vi "数字量输出配置.vi"() -> ()   [LabVIEW 2010]
panel:
  in  "保持输出":bool
  in  "同步_A2":i32
  in  "同步_A1":i32
  in  "数组_输入值":enum16{"0", "1"}[][](array[ring])
  in  "数组_选择?":bool[][](array[boolean])
  in  "btn_置1_5":bool
  in  "btn_置1_4":bool
  in  "btn_置1_3":bool
  in  "btn_置1_2":bool
  in  "btn_全选_5":bool
  in  "btn_全选_4":bool
  in  "btn_全选_3":bool
  in  "btn_全选_2":bool
  in  "btn_置1_1":bool
  in  "btn_全选_1":bool
  in  "CAN端口":u16
  out "light_80":bool
  out "light_79":bool
  out "light_78":bool
  out "light_77":bool
  out "light_76":bool
  out "light_75":bool
  out "light_74":bool
  out "light_73":bool
  out "light_72":bool
  out "light_71":bool
  out "light_70":bool
  out "light_69":bool
  out "light_68":bool
  out "light_67":bool
  out "light_66":bool
  out "light_65":bool
  in  "输入值_73":enum16{"0", "1"}(ring)
  in  "输入值_80":enum16{"0", "1"}(ring)
  in  "输入值_79":enum16{"0", "1"}(ring)
  in  "输入值_78":enum16{"0", "1"}(ring)
  in  "输入值_77":enum16{"0", "1"}(ring)
  in  "输入值_76":enum16{"0", "1"}(ring)
  in  "输入值_75":enum16{"0", "1"}(ring)
  in  "输入值_74":enum16{"0", "1"}(ring)
  in  "输入值_65":enum16{"0", "1"}(ring)
  in  "输入值_72":enum16{"0", "1"}(ring)
  in  "输入值_71":enum16{"0", "1"}(ring)
  in  "输入值_70":enum16{"0", "1"}(ring)
  in  "输入值_69":enum16{"0", "1"}(ring)
  in  "输入值_68":enum16{"0", "1"}(ring)
  in  "输入值_67":enum16{"0", "1"}(ring)
  in  "输入值_66":enum16{"0", "1"}(ring)
  in  "单选_第73路":bool
  in  "单选_第80路":bool
  in  "单选_第79路":bool
  in  "单选_第78路":bool
  in  "单选_第77路":bool
  in  "单选_第76路":bool
  in  "单选_第75路":bool
  in  "单选_第74路":bool
  in  "单选_第65路":bool
  in  "单选_第72路":bool
  in  "单选_第71路":bool
  in  "单选_第70路":bool
  in  "单选_第69路":bool
  in  "单选_第68路":bool
  in  "单选_第67路":bool
  in  "单选_第66路":bool
  out "light_64":bool
  out "light_63":bool
  out "light_62":bool
  out "light_61":bool
  out "light_60":bool
  out "light_59":bool
  out "light_58":bool
  out "light_57":bool
  out "light_56":bool
  out "light_55":bool
  out "light_54":bool
  out "light_53":bool
  out "light_52":bool
  out "light_51":bool
  out "light_50":bool
  out "light_49":bool
  in  "输入值_57":enum16{"0", "1"}(ring)
  in  "输入值_64":enum16{"0", "1"}(ring)
  in  "输入值_63":enum16{"0", "1"}(ring)
  in  "输入值_62":enum16{"0", "1"}(ring)
  in  "输入值_61":enum16{"0", "1"}(ring)
  in  "输入值_60":enum16{"0", "1"}(ring)
  in  "输入值_59":enum16{"0", "1"}(ring)
  in  "输入值_58":enum16{"0", "1"}(ring)
  in  "输入值_49":enum16{"0", "1"}(ring)
  in  "输入值_56":enum16{"0", "1"}(ring)
  in  "输入值_55":enum16{"0", "1"}(ring)
  in  "输入值_54":enum16{"0", "1"}(ring)
  in  "输入值_53":enum16{"0", "1"}(ring)
  in  "输入值_52":enum16{"0", "1"}(ring)
  in  "输入值_51":enum16{"0", "1"}(ring)
  in  "输入值_50":enum16{"0", "1"}(ring)
  in  "单选_第57路":bool
  in  "单选_第64路":bool
  in  "单选_第63路":bool
  in  "单选_第62路":bool
  in  "单选_第61路":bool
  in  "单选_第60路":bool
  in  "单选_第59路":bool
  in  "单选_第58路":bool
  in  "单选_第49路":bool
  in  "单选_第56路":bool
  in  "单选_第55路":bool
  in  "单选_第54路":bool
  in  "单选_第53路":bool
  in  "单选_第52路":bool
  in  "单选_第51路":bool
  in  "单选_第50路":bool
  out "light_48":bool
  out "light_47":bool
  out "light_46":bool
  out "light_45":bool
  out "light_44":bool
  out "light_43":bool
  out "light_42":bool
  out "light_41":bool
  out "light_40":bool
  out "light_39":bool
  out "light_38":bool
  out "light_37":bool
  out "light_36":bool
  out "light_35":bool
  out "light_34":bool
  out "light_33":bool
  in  "输入值_41":enum16{"0", "1"}(ring)
  in  "输入值_48":enum16{"0", "1"}(ring)
  in  "输入值_47":enum16{"0", "1"}(ring)
  in  "输入值_46":enum16{"0", "1"}(ring)
  in  "输入值_45":enum16{"0", "1"}(ring)
  in  "输入值_44":enum16{"0", "1"}(ring)
  in  "输入值_43":enum16{"0", "1"}(ring)
  in  "输入值_42":enum16{"0", "1"}(ring)
  in  "输入值_33":enum16{"0", "1"}(ring)
  in  "输入值_40":enum16{"0", "1"}(ring)
  in  "输入值_39":enum16{"0", "1"}(ring)
  in  "输入值_38":enum16{"0", "1"}(ring)
  in  "输入值_37":enum16{"0", "1"}(ring)
  in  "输入值_36":enum16{"0", "1"}(ring)
  in  "输入值_35":enum16{"0", "1"}(ring)
  in  "输入值_34":enum16{"0", "1"}(ring)
  in  "单选_第41路":bool
  in  "单选_第48路":bool
  in  "单选_第47路":bool
  in  "单选_第46路":bool
  in  "单选_第45路":bool
  in  "单选_第44路":bool
  in  "单选_第43路":bool
  in  "单选_第42路":bool
  in  "单选_第33路":bool
  in  "单选_第40路":bool
  in  "单选_第39路":bool
  in  "单选_第38路":bool
  in  "单选_第37路":bool
  in  "单选_第36路":bool
  in  "单选_第35路":bool
  in  "单选_第34路":bool
  out "light_32":bool
  out "light_31":bool
  out "light_30":bool
  out "light_29":bool
  out "light_28":bool
  out "light_27":bool
  out "light_26":bool
  out "light_25":bool
  out "light_24":bool
  out "light_23":bool
  out "light_22":bool
  out "light_21":bool
  out "light_20":bool
  out "light_19":bool
  out "light_18":bool
  out "light_17":bool
  in  "输入值_25":enum16{"0", "1"}(ring)
  in  "输入值_32":enum16{"0", "1"}(ring)
  in  "输入值_31":enum16{"0", "1"}(ring)
  in  "输入值_30":enum16{"0", "1"}(ring)
  in  "输入值_29":enum16{"0", "1"}(ring)
  in  "输入值_28":enum16{"0", "1"}(ring)
  in  "输入值_27":enum16{"0", "1"}(ring)
  in  "输入值_26":enum16{"0", "1"}(ring)
  in  "输入值_17":enum16{"0", "1"}(ring)
  in  "输入值_24":enum16{"0", "1"}(ring)
  in  "输入值_23":enum16{"0", "1"}(ring)
  in  "输入值_22":enum16{"0", "1"}(ring)
  in  "输入值_21":enum16{"0", "1"}(ring)
  in  "输入值_20":enum16{"0", "1"}(ring)
  in  "输入值_19":enum16{"0", "1"}(ring)
  in  "输入值_18":enum16{"0", "1"}(ring)
  in  "单选_第25路":bool
  in  "单选_第32路":bool
  in  "单选_第31路":bool
  in  "单选_第30路":bool
  in  "单选_第29路":bool
  in  "单选_第28路":bool
  in  "单选_第27路":bool
  in  "单选_第26路":bool
  in  "单选_第17路":bool
  in  "单选_第24路":bool
  in  "单选_第23路":bool
  in  "单选_第22路":bool
  in  "单选_第21路":bool
  in  "单选_第20路":bool
  in  "单选_第19路":bool
  in  "单选_第18路":bool
  in  "D_IN_5":string[][](table) caption="表格"
  in  "D_IN_4":string[][](table) caption="表格"
  in  "D_IN_3":string[][](table) caption="表格"
  in  "D_IN_2":string[][](table) caption="表格"
  out "light_16":bool
  out "light_15":bool
  out "light_14":bool
  out "light_13":bool
  out "light_12":bool
  out "light_11":bool
  out "light_10":bool
  out "light_9":bool
  out "light_8":bool
  out "light_7":bool
  out "light_6":bool
  out "light_5":bool
  out "light_4":bool
  out "light_3":bool
  out "light_2":bool
  out "light_1":bool
  in  "输入值_9":enum16{"0", "1"}(ring)
  in  "输入值_16":enum16{"0", "1"}(ring)
  in  "输入值_15":enum16{"0", "1"}(ring)
  in  "输入值_14":enum16{"0", "1"}(ring)
  in  "输入值_13":enum16{"0", "1"}(ring)
  in  "输入值_12":enum16{"0", "1"}(ring)
  in  "输入值_11":enum16{"0", "1"}(ring)
  in  "输入值_10":enum16{"0", "1"}(ring)
  in  "输入值_1":enum16{"0", "1"}(ring)
  in  "输入值_8":enum16{"0", "1"}(ring)
  in  "输入值_7":enum16{"0", "1"}(ring)
  in  "输入值_6":enum16{"0", "1"}(ring)
  in  "输入值_5":enum16{"0", "1"}(ring)
  in  "输入值_4":enum16{"0", "1"}(ring)
  in  "输入值_3":enum16{"0", "1"}(ring)
  in  "输入值_2":enum16{"0", "1"}(ring)
  in  "单选_第9路":bool
  in  "单选_第16路":bool
  in  "单选_第15路":bool
  in  "单选_第14路":bool
  in  "单选_第13路":bool
  in  "单选_第12路":bool
  in  "单选_第11路":bool
  in  "单选_第10路":bool
  in  "单选_第1路":bool
  in  "单选_第8路":bool
  in  "单选_第7路":bool
  in  "单选_第6路":bool
  in  "单选_第5路":bool
  in  "单选_第4路":bool
  in  "单选_第3路":bool
  in  "单选_第2路":bool
  in  "D_IN_1":string[][](table) caption="表格"
  out "关闭？":bool
  out "测试结论":string
  in  "btn_置0":bool
  in  "btn_置1":bool
  in  "btn_反选":bool
  in  "btn_全选":bool
  in  "btn_关闭":bool
  in  "btn_开始试验":bool
  # "第一组数字量输出"
  # "第二组数字量输出"
  # "第三组数字量输出"
  # "第四组数字量输出(PWM)"
  # "第五组数字量输出(I/O)"
  # "测试结论："
  # "5X16"
  # "5X16"
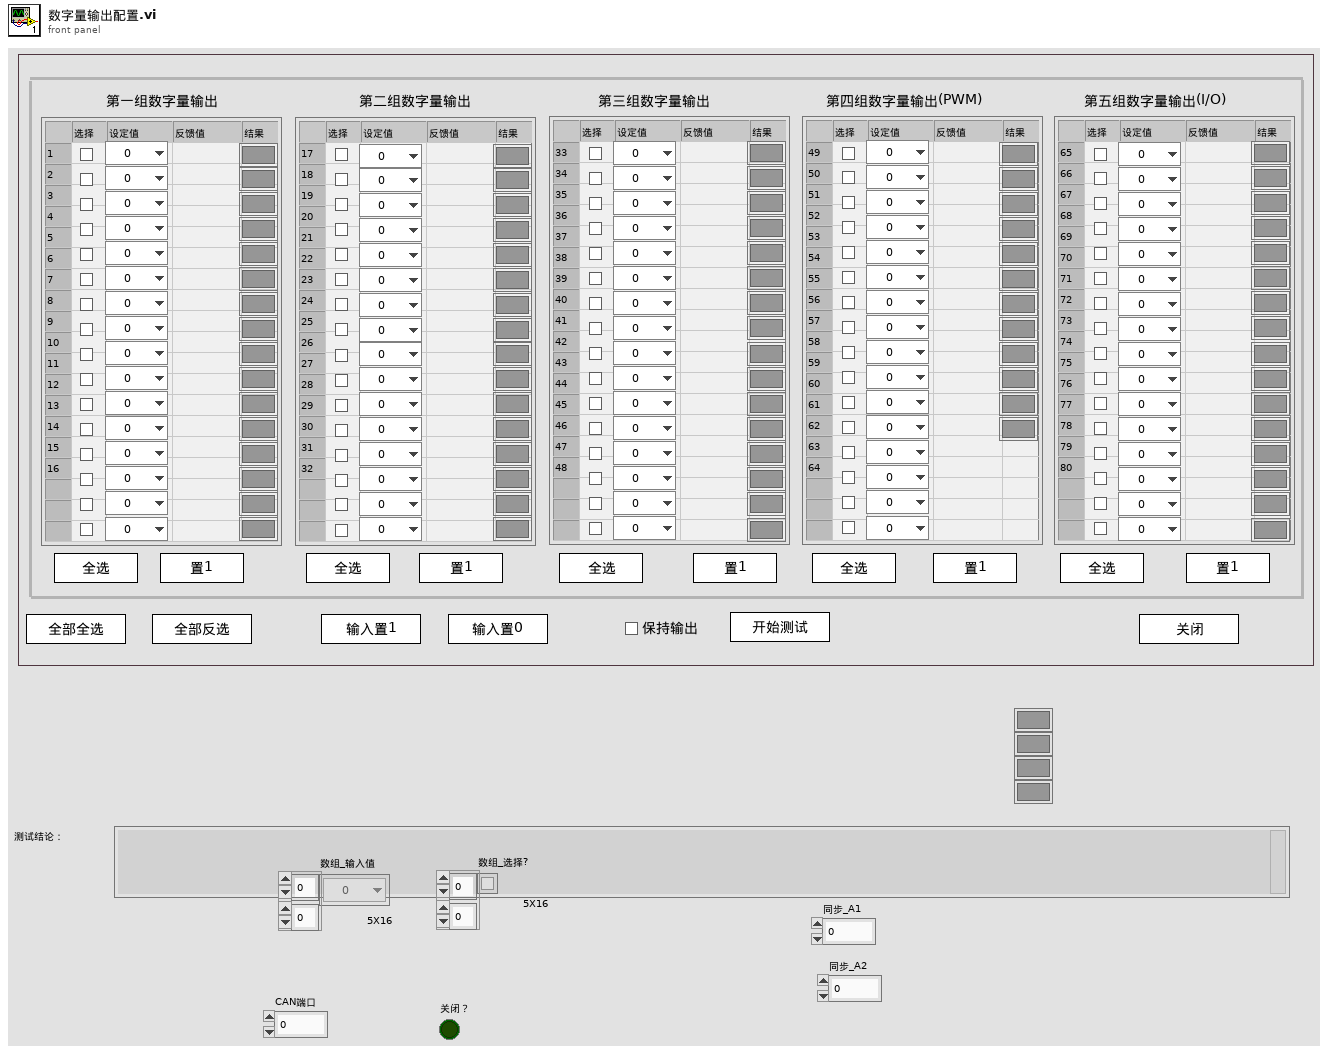
[diagram p1: front panel]
types:
  T1 = enum8{"Enabled", "Disabled", "Disabled and Grayed Out"}
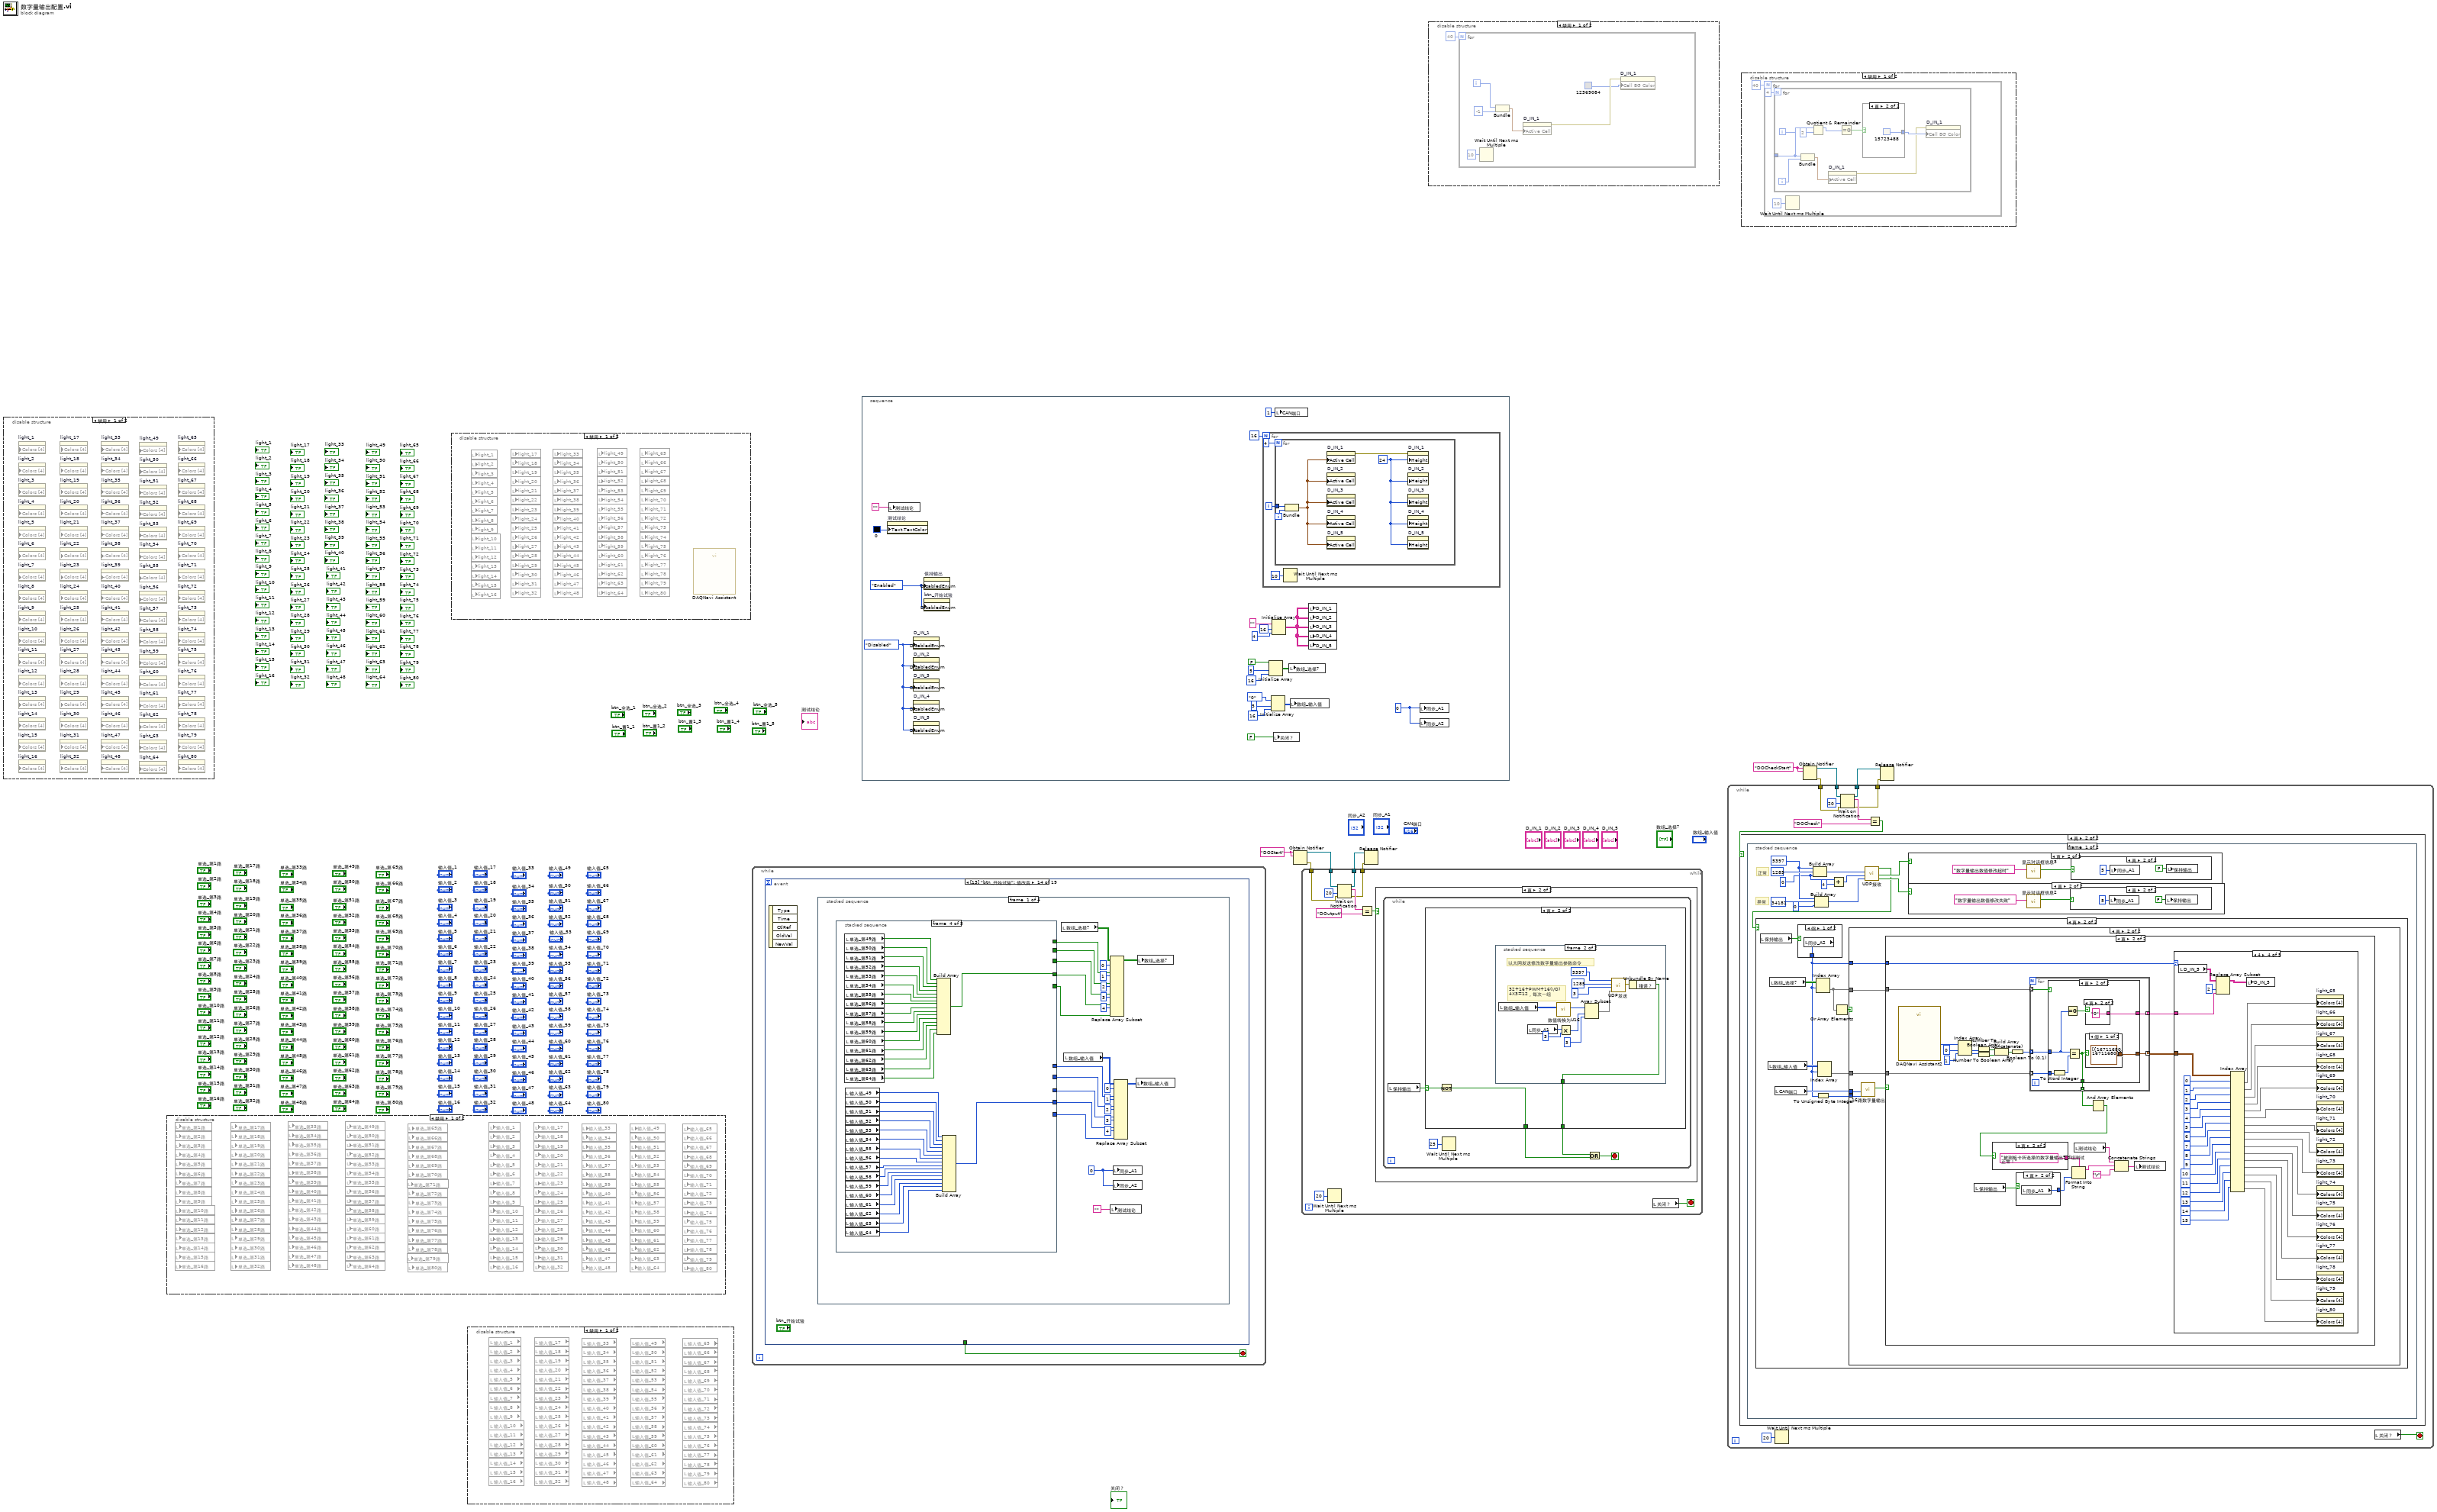
[diagram p0: block diagram]
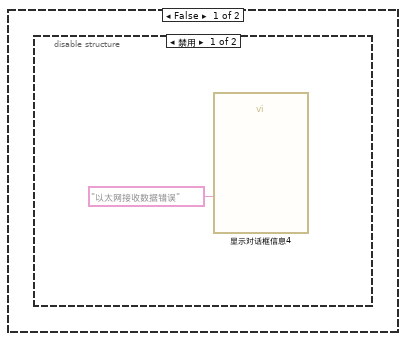
[diagram p7: hidden frame]
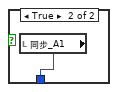
[diagram p9: hidden frame]
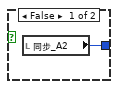
[diagram p12: hidden frame]
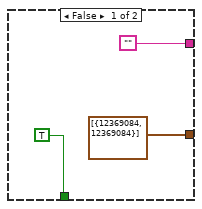
[diagram p13: hidden frame]
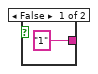
[diagram p14: hidden frame]
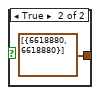
[diagram p15: hidden frame]
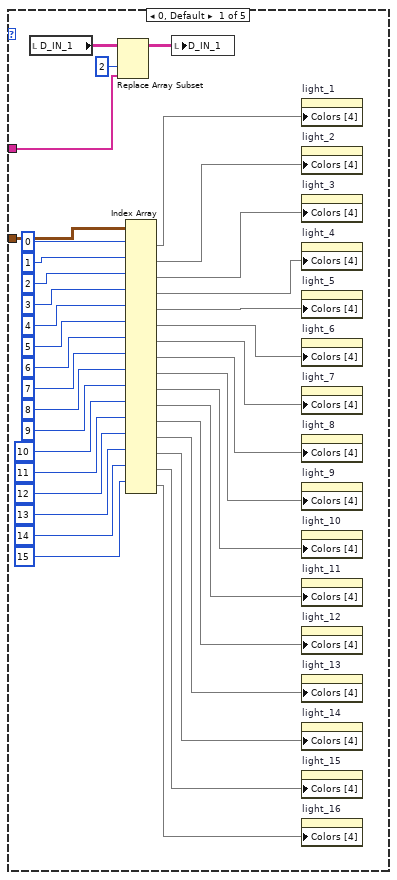
[diagram p16: hidden frame]
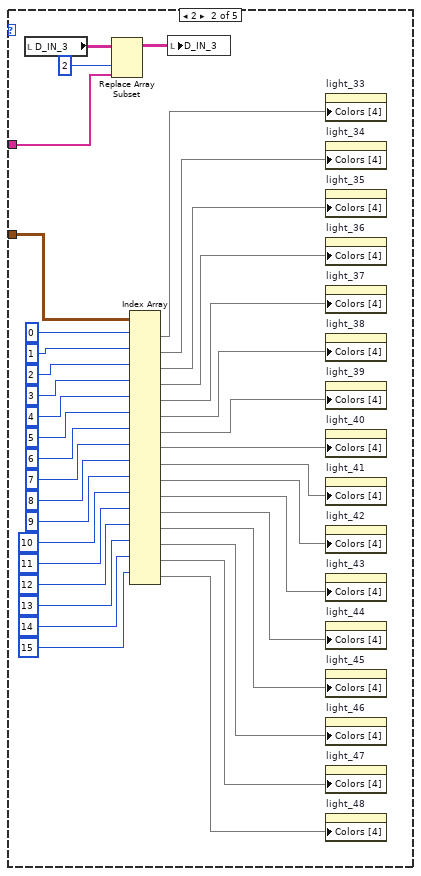
[diagram p17: hidden frame]
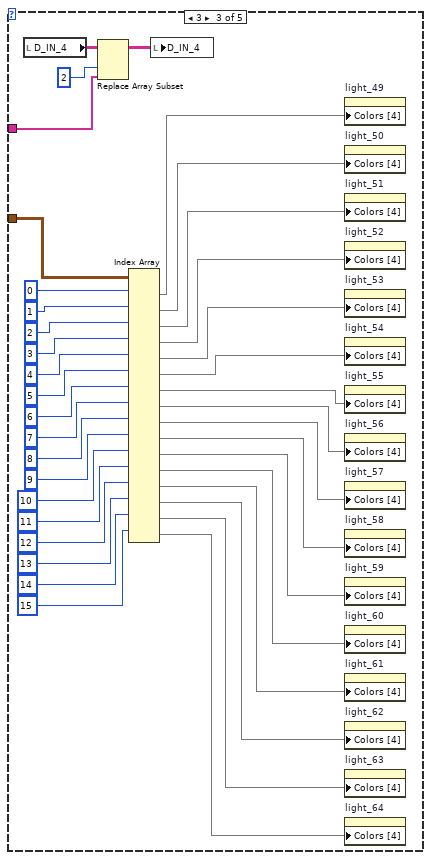
[diagram p18: hidden frame]
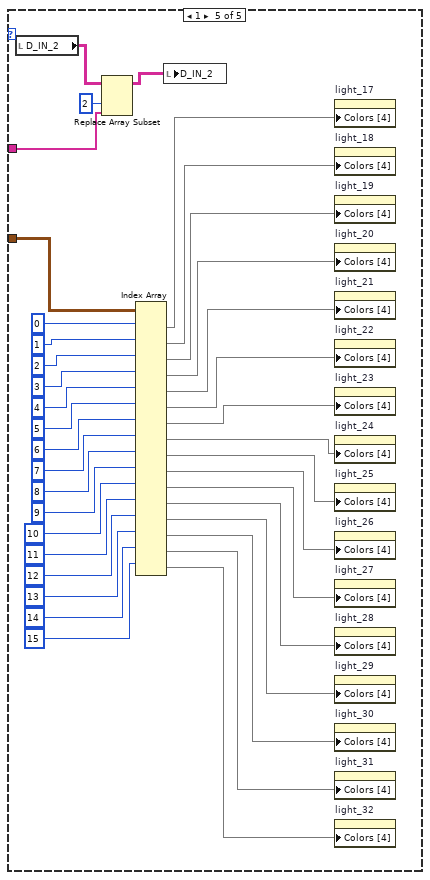
[diagram p19: hidden frame]
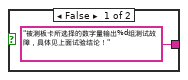
[diagram p20: hidden frame]
diagram:
  w5 = "DOCheckStart" ("名称（未命名）")
  w8 = "DOStart" ("名称（未命名）")
  n1 = disable-structure shown="禁用" {
    frame Disabled {
      n2 = property on="light_1" class="Bool (严格)" props=["Colors [4]"]() -> ()  [unwired: 3 in, 2 out]
      n3 = property on="light_2" class="Bool (严格)" props=["Colors [4]"]() -> ()  [unwired: 3 in, 2 out]
      n4 = property on="light_3" class="Bool (严格)" props=["Colors [4]"]() -> ()  [unwired: 3 in, 2 out]
      n5 = property on="light_4" class="Bool (严格)" props=["Colors [4]"]() -> ()  [unwired: 3 in, 2 out]
      n6 = property on="light_5" class="Bool (严格)" props=["Colors [4]"]() -> ()  [unwired: 3 in, 2 out]
      n7 = property on="light_6" class="Bool (严格)" props=["Colors [4]"]() -> ()  [unwired: 3 in, 2 out]
      n8 = property on="light_7" class="Bool (严格)" props=["Colors [4]"]() -> ()  [unwired: 3 in, 2 out]
      n9 = property on="light_8" class="Bool (严格)" props=["Colors [4]"]() -> ()  [unwired: 3 in, 2 out]
      n10 = property on="light_9" class="Bool (严格)" props=["Colors [4]"]() -> ()  [unwired: 3 in, 2 out]
      n11 = property on="light_10" class="Bool (严格)" props=["Colors [4]"]() -> ()  [unwired: 3 in, 2 out]
      n12 = property on="light_11" class="Bool (严格)" props=["Colors [4]"]() -> ()  [unwired: 3 in, 2 out]
      n13 = property on="light_12" class="Bool (严格)" props=["Colors [4]"]() -> ()  [unwired: 3 in, 2 out]
      n14 = property on="light_13" class="Bool (严格)" props=["Colors [4]"]() -> ()  [unwired: 3 in, 2 out]
      n15 = property on="light_14" class="Bool (严格)" props=["Colors [4]"]() -> ()  [unwired: 3 in, 2 out]
      n16 = property on="light_15" class="Bool (严格)" props=["Colors [4]"]() -> ()  [unwired: 3 in, 2 out]
      n17 = property on="light_16" class="Bool (严格)" props=["Colors [4]"]() -> ()  [unwired: 3 in, 2 out]
      n18 = property on="light_17" class="Bool (严格)" props=["Colors [4]"]() -> ()  [unwired: 3 in, 2 out]
      n19 = property on="light_18" class="Bool (严格)" props=["Colors [4]"]() -> ()  [unwired: 3 in, 2 out]
      n20 = property on="light_19" class="Bool (严格)" props=["Colors [4]"]() -> ()  [unwired: 3 in, 2 out]
      n21 = property on="light_20" class="Bool (严格)" props=["Colors [4]"]() -> ()  [unwired: 3 in, 2 out]
      n22 = property on="light_21" class="Bool (严格)" props=["Colors [4]"]() -> ()  [unwired: 3 in, 2 out]
      n23 = property on="light_22" class="Bool (严格)" props=["Colors [4]"]() -> ()  [unwired: 3 in, 2 out]
      n24 = property on="light_23" class="Bool (严格)" props=["Colors [4]"]() -> ()  [unwired: 3 in, 2 out]
      n25 = property on="light_24" class="Bool (严格)" props=["Colors [4]"]() -> ()  [unwired: 3 in, 2 out]
      n26 = property on="light_25" class="Bool (严格)" props=["Colors [4]"]() -> ()  [unwired: 3 in, 2 out]
      n27 = property on="light_26" class="Bool (严格)" props=["Colors [4]"]() -> ()  [unwired: 3 in, 2 out]
      n28 = property on="light_27" class="Bool (严格)" props=["Colors [4]"]() -> ()  [unwired: 3 in, 2 out]
      n29 = property on="light_28" class="Bool (严格)" props=["Colors [4]"]() -> ()  [unwired: 3 in, 2 out]
      n30 = property on="light_29" class="Bool (严格)" props=["Colors [4]"]() -> ()  [unwired: 3 in, 2 out]
      n31 = property on="light_30" class="Bool (严格)" props=["Colors [4]"]() -> ()  [unwired: 3 in, 2 out]
      n32 = property on="light_31" class="Bool (严格)" props=["Colors [4]"]() -> ()  [unwired: 3 in, 2 out]
      n33 = property on="light_32" class="Bool (严格)" props=["Colors [4]"]() -> ()  [unwired: 3 in, 2 out]
      n34 = property on="light_33" class="Bool (严格)" props=["Colors [4]"]() -> ()  [unwired: 3 in, 2 out]
      n35 = property on="light_34" class="Bool (严格)" props=["Colors [4]"]() -> ()  [unwired: 3 in, 2 out]
      n36 = property on="light_35" class="Bool (严格)" props=["Colors [4]"]() -> ()  [unwired: 3 in, 2 out]
      n37 = property on="light_36" class="Bool (严格)" props=["Colors [4]"]() -> ()  [unwired: 3 in, 2 out]
      n38 = property on="light_37" class="Bool (严格)" props=["Colors [4]"]() -> ()  [unwired: 3 in, 2 out]
      n39 = property on="light_38" class="Bool (严格)" props=["Colors [4]"]() -> ()  [unwired: 3 in, 2 out]
      n40 = property on="light_39" class="Bool (严格)" props=["Colors [4]"]() -> ()  [unwired: 3 in, 2 out]
      n41 = property on="light_40" class="Bool (严格)" props=["Colors [4]"]() -> ()  [unwired: 3 in, 2 out]
      n42 = property on="light_41" class="Bool (严格)" props=["Colors [4]"]() -> ()  [unwired: 3 in, 2 out]
      n43 = property on="light_42" class="Bool (严格)" props=["Colors [4]"]() -> ()  [unwired: 3 in, 2 out]
      n44 = property on="light_43" class="Bool (严格)" props=["Colors [4]"]() -> ()  [unwired: 3 in, 2 out]
      n45 = property on="light_44" class="Bool (严格)" props=["Colors [4]"]() -> ()  [unwired: 3 in, 2 out]
      n46 = property on="light_45" class="Bool (严格)" props=["Colors [4]"]() -> ()  [unwired: 3 in, 2 out]
      n47 = property on="light_46" class="Bool (严格)" props=["Colors [4]"]() -> ()  [unwired: 3 in, 2 out]
      n48 = property on="light_47" class="Bool (严格)" props=["Colors [4]"]() -> ()  [unwired: 3 in, 2 out]
      n49 = property on="light_48" class="Bool (严格)" props=["Colors [4]"]() -> ()  [unwired: 3 in, 2 out]
      n50 = property on="light_49" class="Bool (严格)" props=["Colors [4]"]() -> ()  [unwired: 3 in, 2 out]
      n51 = property on="light_50" class="Bool (严格)" props=["Colors [4]"]() -> ()  [unwired: 3 in, 2 out]
      n52 = property on="light_51" class="Bool (严格)" props=["Colors [4]"]() -> ()  [unwired: 3 in, 2 out]
      n53 = property on="light_52" class="Bool (严格)" props=["Colors [4]"]() -> ()  [unwired: 3 in, 2 out]
      n54 = property on="light_53" class="Bool (严格)" props=["Colors [4]"]() -> ()  [unwired: 3 in, 2 out]
      n55 = property on="light_54" class="Bool (严格)" props=["Colors [4]"]() -> ()  [unwired: 3 in, 2 out]
      n56 = property on="light_55" class="Bool (严格)" props=["Colors [4]"]() -> ()  [unwired: 3 in, 2 out]
      n57 = property on="light_56" class="Bool (严格)" props=["Colors [4]"]() -> ()  [unwired: 3 in, 2 out]
      n58 = property on="light_57" class="Bool (严格)" props=["Colors [4]"]() -> ()  [unwired: 3 in, 2 out]
      n59 = property on="light_58" class="Bool (严格)" props=["Colors [4]"]() -> ()  [unwired: 3 in, 2 out]
      n60 = property on="light_59" class="Bool (严格)" props=["Colors [4]"]() -> ()  [unwired: 3 in, 2 out]
      n61 = property on="light_60" class="Bool (严格)" props=["Colors [4]"]() -> ()  [unwired: 3 in, 2 out]
      n62 = property on="light_61" class="Bool (严格)" props=["Colors [4]"]() -> ()  [unwired: 3 in, 2 out]
      n63 = property on="light_62" class="Bool (严格)" props=["Colors [4]"]() -> ()  [unwired: 3 in, 2 out]
      n64 = property on="light_63" class="Bool (严格)" props=["Colors [4]"]() -> ()  [unwired: 3 in, 2 out]
      n65 = property on="light_64" class="Bool (严格)" props=["Colors [4]"]() -> ()  [unwired: 3 in, 2 out]
      n66 = property on="light_65" class="Bool (严格)" props=["Colors [4]"]() -> ()  [unwired: 3 in, 2 out]
      n67 = property on="light_66" class="Bool (严格)" props=["Colors [4]"]() -> ()  [unwired: 3 in, 2 out]
      n68 = property on="light_67" class="Bool (严格)" props=["Colors [4]"]() -> ()  [unwired: 3 in, 2 out]
      n69 = property on="light_68" class="Bool (严格)" props=["Colors [4]"]() -> ()  [unwired: 3 in, 2 out]
      n70 = property on="light_69" class="Bool (严格)" props=["Colors [4]"]() -> ()  [unwired: 3 in, 2 out]
      n71 = property on="light_70" class="Bool (严格)" props=["Colors [4]"]() -> ()  [unwired: 3 in, 2 out]
      n72 = property on="light_71" class="Bool (严格)" props=["Colors [4]"]() -> ()  [unwired: 3 in, 2 out]
      n73 = property on="light_72" class="Bool (严格)" props=["Colors [4]"]() -> ()  [unwired: 3 in, 2 out]
      n74 = property on="light_73" class="Bool (严格)" props=["Colors [4]"]() -> ()  [unwired: 3 in, 2 out]
      n75 = property on="light_74" class="Bool (严格)" props=["Colors [4]"]() -> ()  [unwired: 3 in, 2 out]
      n76 = property on="light_75" class="Bool (严格)" props=["Colors [4]"]() -> ()  [unwired: 3 in, 2 out]
      n77 = property on="light_76" class="Bool (严格)" props=["Colors [4]"]() -> ()  [unwired: 3 in, 2 out]
      n78 = property on="light_77" class="Bool (严格)" props=["Colors [4]"]() -> ()  [unwired: 3 in, 2 out]
      n79 = property on="light_78" class="Bool (严格)" props=["Colors [4]"]() -> ()  [unwired: 3 in, 2 out]
      n80 = property on="light_79" class="Bool (严格)" props=["Colors [4]"]() -> ()  [unwired: 3 in, 2 out]
      n81 = property on="light_80" class="Bool (严格)" props=["Colors [4]"]() -> ()  [unwired: 3 in, 2 out]
    }
    frame Enabled {
    }
  }
  n82 = disable-structure shown="禁用" {
    frame Disabled {
      n83 = local read "单选_第1路"() -> ()  [unwired: 1 in]
      n84 = local read "单选_第2路"() -> ()  [unwired: 1 in]
      n85 = local read "单选_第3路"() -> ()  [unwired: 1 in]
      n86 = local read "单选_第4路"() -> ()  [unwired: 1 in]
      n87 = local read "单选_第5路"() -> ()  [unwired: 1 in]
      n88 = local read "单选_第6路"() -> ()  [unwired: 1 in]
      n89 = local read "单选_第7路"() -> ()  [unwired: 1 in]
      n90 = local read "单选_第8路"() -> ()  [unwired: 1 in]
      n91 = local read "单选_第9路"() -> ()  [unwired: 1 in]
      n92 = local read "单选_第10路"() -> ()  [unwired: 1 in]
      n93 = local read "单选_第11路"() -> ()  [unwired: 1 in]
      n94 = local read "单选_第12路"() -> ()  [unwired: 1 in]
      n95 = local read "单选_第13路"() -> ()  [unwired: 1 in]
      n96 = local read "单选_第14路"() -> ()  [unwired: 1 in]
      n97 = local read "单选_第15路"() -> ()  [unwired: 1 in]
      n98 = local read "单选_第16路"() -> ()  [unwired: 1 in]
      n99 = local read "单选_第17路"() -> ()  [unwired: 1 in]
      n100 = local read "单选_第18路"() -> ()  [unwired: 1 in]
      n101 = local read "单选_第19路"() -> ()  [unwired: 1 in]
      n102 = local read "单选_第20路"() -> ()  [unwired: 1 in]
      n103 = local read "单选_第21路"() -> ()  [unwired: 1 in]
      n104 = local read "单选_第22路"() -> ()  [unwired: 1 in]
      n105 = local read "单选_第23路"() -> ()  [unwired: 1 in]
      n106 = local read "单选_第24路"() -> ()  [unwired: 1 in]
      n107 = local read "单选_第25路"() -> ()  [unwired: 1 in]
      n108 = local read "单选_第26路"() -> ()  [unwired: 1 in]
      n109 = local read "单选_第27路"() -> ()  [unwired: 1 in]
      n110 = local read "单选_第28路"() -> ()  [unwired: 1 in]
      n111 = local read "单选_第29路"() -> ()  [unwired: 1 in]
      n112 = local read "单选_第30路"() -> ()  [unwired: 1 in]
      n113 = local read "单选_第31路"() -> ()  [unwired: 1 in]
      n114 = local read "单选_第32路"() -> ()  [unwired: 1 in]
      n115 = local read "单选_第33路"() -> ()  [unwired: 1 in]
      n116 = local read "单选_第34路"() -> ()  [unwired: 1 in]
      n117 = local read "单选_第35路"() -> ()  [unwired: 1 in]
      n118 = local read "单选_第36路"() -> ()  [unwired: 1 in]
      n119 = local read "单选_第37路"() -> ()  [unwired: 1 in]
      n120 = local read "单选_第38路"() -> ()  [unwired: 1 in]
      n121 = local read "单选_第39路"() -> ()  [unwired: 1 in]
      n122 = local read "单选_第40路"() -> ()  [unwired: 1 in]
      n123 = local read "单选_第41路"() -> ()  [unwired: 1 in]
      n124 = local read "单选_第42路"() -> ()  [unwired: 1 in]
      n125 = local read "单选_第43路"() -> ()  [unwired: 1 in]
      n126 = local read "单选_第44路"() -> ()  [unwired: 1 in]
      n127 = local read "单选_第45路"() -> ()  [unwired: 1 in]
      n128 = local read "单选_第46路"() -> ()  [unwired: 1 in]
      n129 = local read "单选_第47路"() -> ()  [unwired: 1 in]
      n130 = local read "单选_第48路"() -> ()  [unwired: 1 in]
      n131 = local read "单选_第49路"() -> ()  [unwired: 1 in]
      n132 = local read "单选_第50路"() -> ()  [unwired: 1 in]
      n133 = local read "单选_第51路"() -> ()  [unwired: 1 in]
      n134 = local read "单选_第52路"() -> ()  [unwired: 1 in]
      n135 = local read "单选_第53路"() -> ()  [unwired: 1 in]
      n136 = local read "单选_第54路"() -> ()  [unwired: 1 in]
      n137 = local read "单选_第55路"() -> ()  [unwired: 1 in]
      n138 = local read "单选_第56路"() -> ()  [unwired: 1 in]
      n139 = local read "单选_第57路"() -> ()  [unwired: 1 in]
      n140 = local read "单选_第58路"() -> ()  [unwired: 1 in]
      n141 = local read "单选_第59路"() -> ()  [unwired: 1 in]
      n142 = local read "单选_第60路"() -> ()  [unwired: 1 in]
      n143 = local read "单选_第61路"() -> ()  [unwired: 1 in]
      n144 = local read "单选_第62路"() -> ()  [unwired: 1 in]
      n145 = local read "单选_第63路"() -> ()  [unwired: 1 in]
      n146 = local read "单选_第64路"() -> ()  [unwired: 1 in]
      n147 = local read "单选_第71路"() -> ()  [unwired: 1 in]
      n148 = local read "单选_第79路"() -> ()  [unwired: 1 in]
      n149 = local read "单选_第65路"() -> ()  [unwired: 1 in]
      n150 = local read "单选_第66路"() -> ()  [unwired: 1 in]
      n151 = local read "单选_第67路"() -> ()  [unwired: 1 in]
      n152 = local read "单选_第68路"() -> ()  [unwired: 1 in]
      n153 = local read "单选_第69路"() -> ()  [unwired: 1 in]
      n154 = local read "单选_第70路"() -> ()  [unwired: 1 in]
      n155 = local read "单选_第72路"() -> ()  [unwired: 1 in]
      n156 = local read "单选_第73路"() -> ()  [unwired: 1 in]
      n157 = local read "单选_第74路"() -> ()  [unwired: 1 in]
      n158 = local read "单选_第75路"() -> ()  [unwired: 1 in]
      n159 = local read "单选_第76路"() -> ()  [unwired: 1 in]
      n160 = local read "单选_第77路"() -> ()  [unwired: 1 in]
      n161 = local read "单选_第78路"() -> ()  [unwired: 1 in]
      n162 = local read "单选_第80路"() -> ()  [unwired: 1 in]
      n163 = local read "输入值_1"() -> ()  [unwired: 1 in]
      n164 = local read "输入值_2"() -> ()  [unwired: 1 in]
      n165 = local read "输入值_3"() -> ()  [unwired: 1 in]
      n166 = local read "输入值_4"() -> ()  [unwired: 1 in]
      n167 = local read "输入值_5"() -> ()  [unwired: 1 in]
      n168 = local read "输入值_6"() -> ()  [unwired: 1 in]
      n169 = local read "输入值_7"() -> ()  [unwired: 1 in]
      n170 = local read "输入值_8"() -> ()  [unwired: 1 in]
      n171 = local read "输入值_9"() -> ()  [unwired: 1 in]
      n172 = local read "输入值_10"() -> ()  [unwired: 1 in]
      n173 = local read "输入值_11"() -> ()  [unwired: 1 in]
      n174 = local read "输入值_12"() -> ()  [unwired: 1 in]
      n175 = local read "输入值_13"() -> ()  [unwired: 1 in]
      n176 = local read "输入值_14"() -> ()  [unwired: 1 in]
      n177 = local read "输入值_15"() -> ()  [unwired: 1 in]
      n178 = local read "输入值_16"() -> ()  [unwired: 1 in]
      n179 = local read "输入值_17"() -> ()  [unwired: 1 in]
      n180 = local read "输入值_18"() -> ()  [unwired: 1 in]
      n181 = local read "输入值_19"() -> ()  [unwired: 1 in]
      n182 = local read "输入值_20"() -> ()  [unwired: 1 in]
      n183 = local read "输入值_21"() -> ()  [unwired: 1 in]
      n184 = local read "输入值_22"() -> ()  [unwired: 1 in]
      n185 = local read "输入值_23"() -> ()  [unwired: 1 in]
      n186 = local read "输入值_24"() -> ()  [unwired: 1 in]
      n187 = local read "输入值_25"() -> ()  [unwired: 1 in]
      n188 = local read "输入值_26"() -> ()  [unwired: 1 in]
      n189 = local read "输入值_27"() -> ()  [unwired: 1 in]
      n190 = local read "输入值_28"() -> ()  [unwired: 1 in]
      n191 = local read "输入值_29"() -> ()  [unwired: 1 in]
      n192 = local read "输入值_30"() -> ()  [unwired: 1 in]
      n193 = local read "输入值_31"() -> ()  [unwired: 1 in]
      n194 = local read "输入值_32"() -> ()  [unwired: 1 in]
      n195 = local read "输入值_33"() -> ()  [unwired: 1 in]
      n196 = local read "输入值_34"() -> ()  [unwired: 1 in]
      n197 = local read "输入值_35"() -> ()  [unwired: 1 in]
      n198 = local read "输入值_36"() -> ()  [unwired: 1 in]
      n199 = local read "输入值_37"() -> ()  [unwired: 1 in]
      n200 = local read "输入值_38"() -> ()  [unwired: 1 in]
      n201 = local read "输入值_39"() -> ()  [unwired: 1 in]
      n202 = local read "输入值_40"() -> ()  [unwired: 1 in]
      n203 = local read "输入值_41"() -> ()  [unwired: 1 in]
      n204 = local read "输入值_42"() -> ()  [unwired: 1 in]
      n205 = local read "输入值_43"() -> ()  [unwired: 1 in]
      n206 = local read "输入值_44"() -> ()  [unwired: 1 in]
      n207 = local read "输入值_45"() -> ()  [unwired: 1 in]
      n208 = local read "输入值_46"() -> ()  [unwired: 1 in]
      n209 = local read "输入值_47"() -> ()  [unwired: 1 in]
      n210 = local read "输入值_48"() -> ()  [unwired: 1 in]
      n211 = local read "输入值_49"() -> ()  [unwired: 1 in]
      n212 = local read "输入值_50"() -> ()  [unwired: 1 in]
      n213 = local read "输入值_51"() -> ()  [unwired: 1 in]
      n214 = local read "输入值_52"() -> ()  [unwired: 1 in]
      n215 = local read "输入值_53"() -> ()  [unwired: 1 in]
      n216 = local read "输入值_54"() -> ()  [unwired: 1 in]
      n217 = local read "输入值_55"() -> ()  [unwired: 1 in]
      n218 = local read "输入值_56"() -> ()  [unwired: 1 in]
      n219 = local read "输入值_57"() -> ()  [unwired: 1 in]
      n220 = local read "输入值_58"() -> ()  [unwired: 1 in]
      n221 = local read "输入值_59"() -> ()  [unwired: 1 in]
      n222 = local read "输入值_60"() -> ()  [unwired: 1 in]
      n223 = local read "输入值_61"() -> ()  [unwired: 1 in]
      n224 = local read "输入值_62"() -> ()  [unwired: 1 in]
      n225 = local read "输入值_63"() -> ()  [unwired: 1 in]
      n226 = local read "输入值_64"() -> ()  [unwired: 1 in]
      n227 = local read "输入值_65"() -> ()  [unwired: 1 in]
      n228 = local read "输入值_66"() -> ()  [unwired: 1 in]
      n229 = local read "输入值_67"() -> ()  [unwired: 1 in]
      n230 = local read "输入值_68"() -> ()  [unwired: 1 in]
      n231 = local read "输入值_69"() -> ()  [unwired: 1 in]
      n232 = local read "输入值_70"() -> ()  [unwired: 1 in]
      n233 = local read "输入值_71"() -> ()  [unwired: 1 in]
      n234 = local read "输入值_72"() -> ()  [unwired: 1 in]
      n235 = local read "输入值_73"() -> ()  [unwired: 1 in]
      n236 = local read "输入值_74"() -> ()  [unwired: 1 in]
      n237 = local read "输入值_75"() -> ()  [unwired: 1 in]
      n238 = local read "输入值_76"() -> ()  [unwired: 1 in]
      n239 = local read "输入值_77"() -> ()  [unwired: 1 in]
      n240 = local read "输入值_78"() -> ()  [unwired: 1 in]
      n241 = local read "输入值_79"() -> ()  [unwired: 1 in]
      n242 = local read "输入值_80"() -> ()  [unwired: 1 in]
    }
    frame Enabled {
    }
  }
  n243 = disable-structure shown="禁用" {
    frame Disabled {
      n244 = local read "light_1"() -> ()  [unwired: 1 in]
      n245 = local read "light_2"() -> ()  [unwired: 1 in]
      n246 = local read "light_3"() -> ()  [unwired: 1 in]
      n247 = local read "light_4"() -> ()  [unwired: 1 in]
      n248 = local read "light_5"() -> ()  [unwired: 1 in]
      n249 = local read "light_6"() -> ()  [unwired: 1 in]
      n250 = local read "light_7"() -> ()  [unwired: 1 in]
      n251 = local read "light_8"() -> ()  [unwired: 1 in]
      n252 = local read "light_9"() -> ()  [unwired: 1 in]
      n253 = local read "light_10"() -> ()  [unwired: 1 in]
      n254 = local read "light_11"() -> ()  [unwired: 1 in]
      n255 = local read "light_12"() -> ()  [unwired: 1 in]
      n256 = local read "light_13"() -> ()  [unwired: 1 in]
      n257 = local read "light_14"() -> ()  [unwired: 1 in]
      n258 = local read "light_15"() -> ()  [unwired: 1 in]
      n259 = local read "light_16"() -> ()  [unwired: 1 in]
      n260 = local read "light_17"() -> ()  [unwired: 1 in]
      n261 = local read "light_18"() -> ()  [unwired: 1 in]
      n262 = local read "light_19"() -> ()  [unwired: 1 in]
      n263 = local read "light_20"() -> ()  [unwired: 1 in]
      n264 = local read "light_21"() -> ()  [unwired: 1 in]
      n265 = local read "light_22"() -> ()  [unwired: 1 in]
      n266 = local read "light_23"() -> ()  [unwired: 1 in]
      n267 = local read "light_24"() -> ()  [unwired: 1 in]
      n268 = local read "light_25"() -> ()  [unwired: 1 in]
      n269 = local read "light_26"() -> ()  [unwired: 1 in]
      n270 = local read "light_27"() -> ()  [unwired: 1 in]
      n271 = local read "light_28"() -> ()  [unwired: 1 in]
      n272 = local read "light_29"() -> ()  [unwired: 1 in]
      n273 = local read "light_30"() -> ()  [unwired: 1 in]
      n274 = local read "light_31"() -> ()  [unwired: 1 in]
      n275 = local read "light_32"() -> ()  [unwired: 1 in]
      n276 = local read "light_33"() -> ()  [unwired: 1 in]
      n277 = local read "light_34"() -> ()  [unwired: 1 in]
      n278 = local read "light_35"() -> ()  [unwired: 1 in]
      n279 = local read "light_36"() -> ()  [unwired: 1 in]
      n280 = local read "light_37"() -> ()  [unwired: 1 in]
      n281 = local read "light_38"() -> ()  [unwired: 1 in]
      n282 = local read "light_39"() -> ()  [unwired: 1 in]
      n283 = local read "light_40"() -> ()  [unwired: 1 in]
      n284 = local read "light_41"() -> ()  [unwired: 1 in]
      n285 = local read "light_42"() -> ()  [unwired: 1 in]
      n286 = local read "light_43"() -> ()  [unwired: 1 in]
      n287 = local read "light_44"() -> ()  [unwired: 1 in]
      n288 = local read "light_45"() -> ()  [unwired: 1 in]
      n289 = local read "light_46"() -> ()  [unwired: 1 in]
      n290 = local read "light_47"() -> ()  [unwired: 1 in]
      n291 = local read "light_48"() -> ()  [unwired: 1 in]
      n292 = local read "light_49"() -> ()  [unwired: 1 in]
      n293 = local read "light_50"() -> ()  [unwired: 1 in]
      n294 = local read "light_51"() -> ()  [unwired: 1 in]
      n295 = local read "light_52"() -> ()  [unwired: 1 in]
      n296 = local read "light_53"() -> ()  [unwired: 1 in]
      n297 = local read "light_54"() -> ()  [unwired: 1 in]
      n298 = local read "light_55"() -> ()  [unwired: 1 in]
      n299 = local read "light_56"() -> ()  [unwired: 1 in]
      n300 = local read "light_57"() -> ()  [unwired: 1 in]
      n301 = local read "light_58"() -> ()  [unwired: 1 in]
      n302 = local read "light_59"() -> ()  [unwired: 1 in]
      n303 = local read "light_60"() -> ()  [unwired: 1 in]
      n304 = local read "light_61"() -> ()  [unwired: 1 in]
      n305 = local read "light_62"() -> ()  [unwired: 1 in]
      n306 = local read "light_63"() -> ()  [unwired: 1 in]
      n307 = local read "light_64"() -> ()  [unwired: 1 in]
      n308 = local read "light_65"() -> ()  [unwired: 1 in]
      n309 = local read "light_66"() -> ()  [unwired: 1 in]
      n310 = local read "light_67"() -> ()  [unwired: 1 in]
      n311 = local read "light_68"() -> ()  [unwired: 1 in]
      n312 = local read "light_69"() -> ()  [unwired: 1 in]
      n313 = local read "light_70"() -> ()  [unwired: 1 in]
      n314 = local read "light_71"() -> ()  [unwired: 1 in]
      n315 = local read "light_72"() -> ()  [unwired: 1 in]
      n316 = local read "light_73"() -> ()  [unwired: 1 in]
      n317 = local read "light_74"() -> ()  [unwired: 1 in]
      n318 = local read "light_75"() -> ()  [unwired: 1 in]
      n319 = local read "light_76"() -> ()  [unwired: 1 in]
      n320 = local read "light_77"() -> ()  [unwired: 1 in]
      n321 = local read "light_78"() -> ()  [unwired: 1 in]
      n322 = local read "light_79"() -> ()  [unwired: 1 in]
      n323 = local read "light_80"() -> ()  [unwired: 1 in]
      n324 = call "DAQNavi Assistant"() -> ()  [unwired: 2 in, 18 out]
    }
    frame Enabled {
    }
  }
  n325 = disable-structure shown="禁用" {
    frame Disabled {
      n326 = local read "输入值_1"() -> ()  [unwired: 1 out]
      n327 = local read "输入值_2"() -> ()  [unwired: 1 out]
      n328 = local read "输入值_3"() -> ()  [unwired: 1 out]
      n329 = local read "输入值_4"() -> ()  [unwired: 1 out]
      n330 = local read "输入值_5"() -> ()  [unwired: 1 out]
      n331 = local read "输入值_6"() -> ()  [unwired: 1 out]
      n332 = local read "输入值_7"() -> ()  [unwired: 1 out]
      n333 = local read "输入值_8"() -> ()  [unwired: 1 out]
      n334 = local read "输入值_9"() -> ()  [unwired: 1 out]
      n335 = local read "输入值_10"() -> ()  [unwired: 1 out]
      n336 = local read "输入值_11"() -> ()  [unwired: 1 out]
      n337 = local read "输入值_12"() -> ()  [unwired: 1 out]
      n338 = local read "输入值_13"() -> ()  [unwired: 1 out]
      n339 = local read "输入值_14"() -> ()  [unwired: 1 out]
      n340 = local read "输入值_15"() -> ()  [unwired: 1 out]
      n341 = local read "输入值_16"() -> ()  [unwired: 1 out]
      n342 = local read "输入值_17"() -> ()  [unwired: 1 out]
      n343 = local read "输入值_18"() -> ()  [unwired: 1 out]
      n344 = local read "输入值_19"() -> ()  [unwired: 1 out]
      n345 = local read "输入值_20"() -> ()  [unwired: 1 out]
      n346 = local read "输入值_21"() -> ()  [unwired: 1 out]
      n347 = local read "输入值_22"() -> ()  [unwired: 1 out]
      n348 = local read "输入值_23"() -> ()  [unwired: 1 out]
      n349 = local read "输入值_24"() -> ()  [unwired: 1 out]
      n350 = local read "输入值_25"() -> ()  [unwired: 1 out]
      n351 = local read "输入值_26"() -> ()  [unwired: 1 out]
      n352 = local read "输入值_27"() -> ()  [unwired: 1 out]
      n353 = local read "输入值_28"() -> ()  [unwired: 1 out]
      n354 = local read "输入值_29"() -> ()  [unwired: 1 out]
      n355 = local read "输入值_30"() -> ()  [unwired: 1 out]
      n356 = local read "输入值_31"() -> ()  [unwired: 1 out]
      n357 = local read "输入值_32"() -> ()  [unwired: 1 out]
      n358 = local read "输入值_33"() -> ()  [unwired: 1 out]
      n359 = local read "输入值_34"() -> ()  [unwired: 1 out]
      n360 = local read "输入值_35"() -> ()  [unwired: 1 out]
      n361 = local read "输入值_36"() -> ()  [unwired: 1 out]
      n362 = local read "输入值_37"() -> ()  [unwired: 1 out]
      n363 = local read "输入值_38"() -> ()  [unwired: 1 out]
      n364 = local read "输入值_39"() -> ()  [unwired: 1 out]
      n365 = local read "输入值_40"() -> ()  [unwired: 1 out]
      n366 = local read "输入值_41"() -> ()  [unwired: 1 out]
      n367 = local read "输入值_42"() -> ()  [unwired: 1 out]
      n368 = local read "输入值_43"() -> ()  [unwired: 1 out]
      n369 = local read "输入值_44"() -> ()  [unwired: 1 out]
      n370 = local read "输入值_45"() -> ()  [unwired: 1 out]
      n371 = local read "输入值_46"() -> ()  [unwired: 1 out]
      n372 = local read "输入值_47"() -> ()  [unwired: 1 out]
      n373 = local read "输入值_48"() -> ()  [unwired: 1 out]
      n374 = local read "输入值_49"() -> ()  [unwired: 1 out]
      n375 = local read "输入值_50"() -> ()  [unwired: 1 out]
      n376 = local read "输入值_51"() -> ()  [unwired: 1 out]
      n377 = local read "输入值_52"() -> ()  [unwired: 1 out]
      n378 = local read "输入值_53"() -> ()  [unwired: 1 out]
      n379 = local read "输入值_54"() -> ()  [unwired: 1 out]
      n380 = local read "输入值_55"() -> ()  [unwired: 1 out]
      n381 = local read "输入值_56"() -> ()  [unwired: 1 out]
      n382 = local read "输入值_57"() -> ()  [unwired: 1 out]
      n383 = local read "输入值_58"() -> ()  [unwired: 1 out]
      n384 = local read "输入值_59"() -> ()  [unwired: 1 out]
      n385 = local read "输入值_60"() -> ()  [unwired: 1 out]
      n386 = local read "输入值_61"() -> ()  [unwired: 1 out]
      n387 = local read "输入值_62"() -> ()  [unwired: 1 out]
      n388 = local read "输入值_63"() -> ()  [unwired: 1 out]
      n389 = local read "输入值_64"() -> ()  [unwired: 1 out]
      n390 = local read "输入值_65"() -> ()  [unwired: 1 out]
      n391 = local read "输入值_66"() -> ()  [unwired: 1 out]
      n392 = local read "输入值_67"() -> ()  [unwired: 1 out]
      n393 = local read "输入值_68"() -> ()  [unwired: 1 out]
      n394 = local read "输入值_69"() -> ()  [unwired: 1 out]
      n395 = local read "输入值_70"() -> ()  [unwired: 1 out]
      n396 = local read "输入值_71"() -> ()  [unwired: 1 out]
      n397 = local read "输入值_72"() -> ()  [unwired: 1 out]
      n398 = local read "输入值_73"() -> ()  [unwired: 1 out]
      n399 = local read "输入值_74"() -> ()  [unwired: 1 out]
      n400 = local read "输入值_75"() -> ()  [unwired: 1 out]
      n401 = local read "输入值_76"() -> ()  [unwired: 1 out]
      n402 = local read "输入值_77"() -> ()  [unwired: 1 out]
      n403 = local read "输入值_78"() -> ()  [unwired: 1 out]
      n404 = local read "输入值_79"() -> ()  [unwired: 1 out]
      n405 = local read "输入值_80"() -> ()  [unwired: 1 out]
    }
    frame Enabled {
    }
  }
  n406 = while {
    stop <- w11 stop-if-true
    n407 = event shown="[13] \"btn_开始试验\": 值改变" {
      selector: _ -> [_ _ _ _ _ _ _ _ _ _ _ _ _ _ _ _ _ _ _]
      dyn-events: _ -> [_ _ _ _ _ _ _ _ _ _ _ _ _ _ _ _ _ _ _]
      timeout: _ -> [_ _ _ _ _ _ _ _ _ _ _ _ _ _ _ _ _ _ _]
      tunnel: [_ w12 w13 _ _ _ _ _ _ _ _ _ _ _ _ _ _ _ _] -> w11
      event Timeout {
        n408 = event-data() -> ()  [unwired: 1 in, 2 out]
      }
      event Panel Close {
        w12 = TRUE ("关闭？")
        n409 = event-data() -> ()  [unwired: 1 in, 3 out]
        n410 = local write "关闭？"(w12) -> ()
      }
      event "btn_关闭": Value Change {
        w13 = TRUE
        n411 = event-data() -> ()  [unwired: 1 in, 5 out]
        n412 = local write "关闭？"(w13) -> ()
      }
      event "btn_全选_1": Value Change {
        n413 = event-data() -> ("NewVal"=w15:bool)  [unwired: 1 in, 4 out]
        n414 = case shown="假" w15 {
          tunnel: [FALSE ("单选_第41路") TRUE ("单选_第41路")] -> w14
          frame False {
          }
          frame True {
          }
        }
        n415 = local write "单选_第1路"(w14) -> ()
        n416 = local write "单选_第2路"(w14) -> ()
        n417 = local write "单选_第3路"(w14) -> ()
        n418 = local write "单选_第4路"(w14) -> ()
        n419 = local write "单选_第5路"(w14) -> ()
        n420 = local write "单选_第6路"(w14) -> ()
        n421 = local write "单选_第7路"(w14) -> ()
        n422 = local write "单选_第8路"(w14) -> ()
        n423 = local write "单选_第9路"(w14) -> ()
        n424 = local write "单选_第10路"(w14) -> ()
        n425 = local write "单选_第11路"(w14) -> ()
        n426 = local write "单选_第12路"(w14) -> ()
        n427 = local write "单选_第13路"(w14) -> ()
        n428 = local write "单选_第14路"(w14) -> ()
        n429 = local write "单选_第15路"(w14) -> ()
        n430 = local write "单选_第16路"(w14) -> ()
      }
      event "btn_全选_2": Value Change {
        n431 = event-data() -> ("NewVal"=w19:bool)  [unwired: 1 in, 4 out]
        n432 = case shown="假" w19 {
          tunnel: [FALSE ("单选_第41路") TRUE ("单选_第41路")] -> w18
          frame False {
          }
          frame True {
          }
        }
        n433 = local write "单选_第17路"(w18) -> ()
        n434 = local write "单选_第18路"(w18) -> ()
        n435 = local write "单选_第19路"(w18) -> ()
        n436 = local write "单选_第20路"(w18) -> ()
        n437 = local write "单选_第21路"(w18) -> ()
        n438 = local write "单选_第22路"(w18) -> ()
        n439 = local write "单选_第23路"(w18) -> ()
        n440 = local write "单选_第24路"(w18) -> ()
        n441 = local write "单选_第25路"(w18) -> ()
        n442 = local write "单选_第26路"(w18) -> ()
        n443 = local write "单选_第27路"(w18) -> ()
        n444 = local write "单选_第28路"(w18) -> ()
        n445 = local write "单选_第29路"(w18) -> ()
        n446 = local write "单选_第30路"(w18) -> ()
        n447 = local write "单选_第31路"(w18) -> ()
        n448 = local write "单选_第32路"(w18) -> ()
      }
      event "btn_全选_3": Value Change {
        n449 = event-data() -> ("NewVal"=w23:bool)  [unwired: 1 in, 4 out]
        n450 = case shown="假" w23 {
          tunnel: [FALSE ("单选_第41路") TRUE ("单选_第41路")] -> w22
          frame False {
          }
          frame True {
          }
        }
        n451 = local write "单选_第33路"(w22) -> ()
        n452 = local write "单选_第34路"(w22) -> ()
        n453 = local write "单选_第35路"(w22) -> ()
        n454 = local write "单选_第36路"(w22) -> ()
        n455 = local write "单选_第37路"(w22) -> ()
        n456 = local write "单选_第38路"(w22) -> ()
        n457 = local write "单选_第39路"(w22) -> ()
        n458 = local write "单选_第40路"(w22) -> ()
        n459 = local write "单选_第41路"(w22) -> ()
        n460 = local write "单选_第42路"(w22) -> ()
        n461 = local write "单选_第43路"(w22) -> ()
        n462 = local write "单选_第44路"(w22) -> ()
        n463 = local write "单选_第45路"(w22) -> ()
        n464 = local write "单选_第46路"(w22) -> ()
        n465 = local write "单选_第47路"(w22) -> ()
        n466 = local write "单选_第48路"(w22) -> ()
      }
      event "btn_全选_4": Value Change {
        n467 = event-data() -> ("NewVal"=w27:bool)  [unwired: 1 in, 4 out]
        n468 = case shown="假" w27 {
          tunnel: [FALSE ("单选_第41路") TRUE ("单选_第41路")] -> w26
          frame False {
          }
          frame True {
          }
        }
        n469 = local write "单选_第49路"(w26) -> ()
        n470 = local write "单选_第50路"(w26) -> ()
        n471 = local write "单选_第51路"(w26) -> ()
        n472 = local write "单选_第52路"(w26) -> ()
        n473 = local write "单选_第53路"(w26) -> ()
        n474 = local write "单选_第54路"(w26) -> ()
        n475 = local write "单选_第55路"(w26) -> ()
        n476 = local write "单选_第56路"(w26) -> ()
        n477 = local write "单选_第57路"(w26) -> ()
        n478 = local write "单选_第58路"(w26) -> ()
        n479 = local write "单选_第59路"(w26) -> ()
        n480 = local write "单选_第60路"(w26) -> ()
        n481 = local write "单选_第61路"(w26) -> ()
        n482 = local write "单选_第62路"(w26) -> ()
        n483 = local write "单选_第63路"(w26) -> ()
        n484 = local write "单选_第64路"(w26) -> ()
      }
      event "btn_全选_5": Value Change {
        n485 = event-data() -> ("NewVal"=w31:bool)  [unwired: 1 in, 4 out]
        n486 = case shown="假" w31 {
          tunnel: [FALSE ("单选_第41路") TRUE ("单选_第41路")] -> w30
          frame False {
          }
          frame True {
          }
        }
        n487 = local write "单选_第71路"(w30) -> ()
        n488 = local write "单选_第79路"(w30) -> ()
        n489 = local write "单选_第65路"(w30) -> ()
        n490 = local write "单选_第66路"(w30) -> ()
        n491 = local write "单选_第67路"(w30) -> ()
        n492 = local write "单选_第68路"(w30) -> ()
        n493 = local write "单选_第69路"(w30) -> ()
        n494 = local write "单选_第70路"(w30) -> ()
        n495 = local write "单选_第72路"(w30) -> ()
        n496 = local write "单选_第73路"(w30) -> ()
        n497 = local write "单选_第74路"(w30) -> ()
        n498 = local write "单选_第75路"(w30) -> ()
        n499 = local write "单选_第76路"(w30) -> ()
        n500 = local write "单选_第77路"(w30) -> ()
        n501 = local write "单选_第78路"(w30) -> ()
        n502 = local write "单选_第80路"(w30) -> ()
      }
      event "btn_置1_1": Value Change {
        n503 = event-data() -> ("NewVal"=w35:bool)  [unwired: 1 in, 4 out]
        n504 = case shown="假" w35 {
          tunnel: [enum16{"0", "1"}."0" ("输入值_41") enum16{"0", "1"}."1" ("输入值_41")] -> w34
          frame False {
          }
          frame True {
          }
        }
        n505 = local write "输入值_1"(w34) -> ()
        n506 = local write "输入值_2"(w34) -> ()
        n507 = local write "输入值_3"(w34) -> ()
        n508 = local write "输入值_4"(w34) -> ()
        n509 = local write "输入值_5"(w34) -> ()
        n510 = local write "输入值_6"(w34) -> ()
        n511 = local write "输入值_7"(w34) -> ()
        n512 = local write "输入值_8"(w34) -> ()
        n513 = local write "输入值_9"(w34) -> ()
        n514 = local write "输入值_10"(w34) -> ()
        n515 = local write "输入值_11"(w34) -> ()
        n516 = local write "输入值_12"(w34) -> ()
        n517 = local write "输入值_13"(w34) -> ()
        n518 = local write "输入值_14"(w34) -> ()
        n519 = local write "输入值_15"(w34) -> ()
        n520 = local write "输入值_16"(w34) -> ()
      }
      event "btn_置1_2": Value Change {
        n521 = event-data() -> ("NewVal"=w39:bool)  [unwired: 1 in, 4 out]
        n522 = case shown="假" w39 {
          tunnel: [enum16{"0", "1"}."0" ("输入值_41") enum16{"0", "1"}."1" ("输入值_41")] -> w38
          frame False {
          }
          frame True {
          }
        }
        n523 = local write "输入值_17"(w38) -> ()
        n524 = local write "输入值_18"(w38) -> ()
        n525 = local write "输入值_19"(w38) -> ()
        n526 = local write "输入值_20"(w38) -> ()
        n527 = local write "输入值_21"(w38) -> ()
        n528 = local write "输入值_22"(w38) -> ()
        n529 = local write "输入值_23"(w38) -> ()
        n530 = local write "输入值_24"(w38) -> ()
        n531 = local write "输入值_25"(w38) -> ()
        n532 = local write "输入值_26"(w38) -> ()
        n533 = local write "输入值_27"(w38) -> ()
        n534 = local write "输入值_28"(w38) -> ()
        n535 = local write "输入值_29"(w38) -> ()
        n536 = local write "输入值_30"(w38) -> ()
        n537 = local write "输入值_31"(w38) -> ()
        n538 = local write "输入值_32"(w38) -> ()
      }
      event "btn_置1_3": Value Change {
        n539 = event-data() -> ("NewVal"=w43:bool)  [unwired: 1 in, 4 out]
        n540 = case shown="假" w43 {
          tunnel: [enum16{"0", "1"}."0" ("输入值_41") enum16{"0", "1"}."1" ("输入值_41")] -> w42
          frame False {
          }
          frame True {
          }
        }
        n541 = local write "输入值_33"(w42) -> ()
        n542 = local write "输入值_34"(w42) -> ()
        n543 = local write "输入值_35"(w42) -> ()
        n544 = local write "输入值_36"(w42) -> ()
        n545 = local write "输入值_37"(w42) -> ()
        n546 = local write "输入值_38"(w42) -> ()
        n547 = local write "输入值_39"(w42) -> ()
        n548 = local write "输入值_40"(w42) -> ()
        n549 = local write "输入值_41"(w42) -> ()
        n550 = local write "输入值_42"(w42) -> ()
        n551 = local write "输入值_43"(w42) -> ()
        n552 = local write "输入值_44"(w42) -> ()
        n553 = local write "输入值_45"(w42) -> ()
        n554 = local write "输入值_46"(w42) -> ()
        n555 = local write "输入值_47"(w42) -> ()
        n556 = local write "输入值_48"(w42) -> ()
      }
      event "btn_置1_4": Value Change {
        n557 = event-data() -> ("NewVal"=w47:bool)  [unwired: 1 in, 4 out]
        n558 = case shown="假" w47 {
          tunnel: [enum16{"0", "1"}."0" ("输入值_41") enum16{"0", "1"}."1" ("输入值_41")] -> w46
          frame False {
          }
          frame True {
          }
        }
        n559 = local write "输入值_49"(w46) -> ()
        n560 = local write "输入值_50"(w46) -> ()
        n561 = local write "输入值_51"(w46) -> ()
        n562 = local write "输入值_52"(w46) -> ()
        n563 = local write "输入值_53"(w46) -> ()
        n564 = local write "输入值_54"(w46) -> ()
        n565 = local write "输入值_55"(w46) -> ()
        n566 = local write "输入值_56"(w46) -> ()
        n567 = local write "输入值_57"(w46) -> ()
        n568 = local write "输入值_58"(w46) -> ()
        n569 = local write "输入值_59"(w46) -> ()
        n570 = local write "输入值_60"(w46) -> ()
        n571 = local write "输入值_61"(w46) -> ()
        n572 = local write "输入值_62"(w46) -> ()
        n573 = local write "输入值_63"(w46) -> ()
        n574 = local write "输入值_64"(w46) -> ()
      }
      event "btn_置1_5": Value Change {
        n575 = event-data() -> ("NewVal"=w51:bool)  [unwired: 1 in, 4 out]
        n576 = case shown="假" w51 {
          tunnel: [enum16{"0", "1"}."0" ("输入值_41") enum16{"0", "1"}."1" ("输入值_41")] -> w50
          frame False {
          }
          frame True {
          }
        }
        n577 = local write "输入值_65"(w50) -> ()
        n578 = local write "输入值_66"(w50) -> ()
        n579 = local write "输入值_67"(w50) -> ()
        n580 = local write "输入值_68"(w50) -> ()
        n581 = local write "输入值_69"(w50) -> ()
        n582 = local write "输入值_70"(w50) -> ()
        n583 = local write "输入值_71"(w50) -> ()
        n584 = local write "输入值_72"(w50) -> ()
        n585 = local write "输入值_73"(w50) -> ()
        n586 = local write "输入值_74"(w50) -> ()
        n587 = local write "输入值_75"(w50) -> ()
        n588 = local write "输入值_76"(w50) -> ()
        n589 = local write "输入值_77"(w50) -> ()
        n590 = local write "输入值_78"(w50) -> ()
        n591 = local write "输入值_79"(w50) -> ()
        n592 = local write "输入值_80"(w50) -> ()
      }
      event "btn_开始试验": Value Change {
        n593 = event-data() -> ()  [unwired: 1 in, 5 out]
        n594 = stacked-sequence {
          frame #0 {
            w55 = 0 ("同步_A1")
            n595 = stacked-sequence {
              tunnel: [w81 _ _ _ _] -> w77
              tunnel: [w80 _ _ _ _] -> w61
              tunnel: [_ w115 _ _ _] -> w75
              tunnel: [_ w114 _ _ _] -> w60
              tunnel: [_ _ w149 _ _] -> w73
              tunnel: [_ _ w148 _ _] -> w59
              tunnel: [_ _ _ w183 _] -> w71
              tunnel: [_ _ _ w182 _] -> w58
              tunnel: [_ _ _ _ w217] -> w69
              tunnel: [_ _ _ _ w216] -> w57
              frame #0 {
                n596 = local read "单选_第1路"() -> (w98:bool)
                n597 = local read "单选_第2路"() -> (w99:bool)
                n598 = local read "单选_第3路"() -> (w100:bool)
                n599 = local read "单选_第4路"() -> (w101:bool)
                n600 = local read "单选_第5路"() -> (w102:bool)
                n601 = local read "单选_第6路"() -> (w103:bool)
                n602 = local read "单选_第7路"() -> (w104:bool)
                n603 = local read "单选_第8路"() -> (w105:bool)
                n604 = local read "单选_第9路"() -> (w106:bool)
                n605 = local read "单选_第10路"() -> (w107:bool)
                n606 = local read "单选_第11路"() -> (w108:bool)
                n607 = local read "单选_第12路"() -> (w109:bool)
                n608 = local read "单选_第13路"() -> (w110:bool)
                n609 = local read "单选_第14路"() -> (w111:bool)
                n610 = local read "单选_第15路"() -> (w112:bool)
                n611 = local read "单选_第16路"() -> (w113:bool)
                n612 = local read "输入值_1"() -> (w82:enum16{"0", "1"})
                n613 = local read "输入值_2"() -> (w83:enum16{"0", "1"})
                n614 = local read "输入值_3"() -> (w84:enum16{"0", "1"})
                n615 = local read "输入值_4"() -> (w85:enum16{"0", "1"})
                n616 = local read "输入值_5"() -> (w86:enum16{"0", "1"})
                n617 = local read "输入值_6"() -> (w87:enum16{"0", "1"})
                n618 = local read "输入值_7"() -> (w88:enum16{"0", "1"})
                n619 = local read "输入值_8"() -> (w89:enum16{"0", "1"})
                n620 = local read "输入值_9"() -> (w90:enum16{"0", "1"})
                n621 = local read "输入值_10"() -> (w91:enum16{"0", "1"})
                n622 = local read "输入值_11"() -> (w92:enum16{"0", "1"})
                n623 = local read "输入值_12"() -> (w93:enum16{"0", "1"})
                n624 = local read "输入值_13"() -> (w94:enum16{"0", "1"})
                n625 = local read "输入值_14"() -> (w95:enum16{"0", "1"})
                n626 = local read "输入值_15"() -> (w96:enum16{"0", "1"})
                n627 = local read "输入值_16"() -> (w97:enum16{"0", "1"})
                n628 = Build Array(w98, w99, w100, w101, w102, w103, w104, w105, w106, w107, w108, w109, w110, w111, w112, w113) -> (w81:bool[])
                n629 = Build Array(w82, w83, w84, w85, w86, w87, w88, w89, w90, w91, w92, w93, w94, w95, w96, w97) -> (w80:enum16{"0", "1"}[])
              }
              frame #1 {
                n630 = local read "单选_第17路"() -> (w132:bool)
                n631 = local read "单选_第18路"() -> (w133:bool)
                n632 = local read "单选_第19路"() -> (w134:bool)
                n633 = local read "单选_第20路"() -> (w135:bool)
                n634 = local read "单选_第21路"() -> (w136:bool)
                n635 = local read "单选_第22路"() -> (w137:bool)
                n636 = local read "单选_第23路"() -> (w138:bool)
                n637 = local read "单选_第24路"() -> (w139:bool)
                n638 = local read "单选_第25路"() -> (w140:bool)
                n639 = local read "单选_第26路"() -> (w141:bool)
                n640 = local read "单选_第27路"() -> (w142:bool)
                n641 = local read "单选_第28路"() -> (w143:bool)
                n642 = local read "单选_第29路"() -> (w144:bool)
                n643 = local read "单选_第30路"() -> (w145:bool)
                n644 = local read "单选_第31路"() -> (w146:bool)
                n645 = local read "单选_第32路"() -> (w147:bool)
                n646 = local read "输入值_17"() -> (w116:enum16{"0", "1"})
                n647 = local read "输入值_18"() -> (w117:enum16{"0", "1"})
                n648 = local read "输入值_19"() -> (w118:enum16{"0", "1"})
                n649 = local read "输入值_20"() -> (w119:enum16{"0", "1"})
                n650 = local read "输入值_21"() -> (w120:enum16{"0", "1"})
                n651 = local read "输入值_22"() -> (w121:enum16{"0", "1"})
                n652 = local read "输入值_23"() -> (w122:enum16{"0", "1"})
                n653 = local read "输入值_24"() -> (w123:enum16{"0", "1"})
                n654 = local read "输入值_25"() -> (w124:enum16{"0", "1"})
                n655 = local read "输入值_26"() -> (w125:enum16{"0", "1"})
                n656 = local read "输入值_27"() -> (w126:enum16{"0", "1"})
                n657 = local read "输入值_28"() -> (w127:enum16{"0", "1"})
                n658 = local read "输入值_29"() -> (w128:enum16{"0", "1"})
                n659 = local read "输入值_30"() -> (w129:enum16{"0", "1"})
                n660 = local read "输入值_31"() -> (w130:enum16{"0", "1"})
                n661 = local read "输入值_32"() -> (w131:enum16{"0", "1"})
                n662 = Build Array(w132, w133, w134, w135, w136, w137, w138, w139, w140, w141, w142, w143, w144, w145, w146, w147) -> (w115:bool[])
                n663 = Build Array(w116, w117, w118, w119, w120, w121, w122, w123, w124, w125, w126, w127, w128, w129, w130, w131) -> (w114:enum16{"0", "1"}[])
              }
              frame #2 {
                n664 = local read "单选_第33路"() -> (w166:bool)
                n665 = local read "单选_第34路"() -> (w167:bool)
                n666 = local read "单选_第35路"() -> (w168:bool)
                n667 = local read "单选_第36路"() -> (w169:bool)
                n668 = local read "单选_第37路"() -> (w170:bool)
                n669 = local read "单选_第38路"() -> (w171:bool)
                n670 = local read "单选_第39路"() -> (w172:bool)
                n671 = local read "单选_第40路"() -> (w173:bool)
                n672 = local read "单选_第41路"() -> (w174:bool)
                n673 = local read "单选_第42路"() -> (w175:bool)
                n674 = local read "单选_第43路"() -> (w176:bool)
                n675 = local read "单选_第44路"() -> (w177:bool)
                n676 = local read "单选_第45路"() -> (w178:bool)
                n677 = local read "单选_第46路"() -> (w179:bool)
                n678 = local read "单选_第47路"() -> (w180:bool)
                n679 = local read "单选_第48路"() -> (w181:bool)
                n680 = local read "输入值_33"() -> (w150:enum16{"0", "1"})
                n681 = local read "输入值_34"() -> (w151:enum16{"0", "1"})
                n682 = local read "输入值_35"() -> (w152:enum16{"0", "1"})
                n683 = local read "输入值_36"() -> (w153:enum16{"0", "1"})
                n684 = local read "输入值_37"() -> (w154:enum16{"0", "1"})
                n685 = local read "输入值_38"() -> (w155:enum16{"0", "1"})
                n686 = local read "输入值_39"() -> (w156:enum16{"0", "1"})
                n687 = local read "输入值_40"() -> (w157:enum16{"0", "1"})
                n688 = local read "输入值_41"() -> (w158:enum16{"0", "1"})
                n689 = local read "输入值_42"() -> (w159:enum16{"0", "1"})
                n690 = local read "输入值_43"() -> (w160:enum16{"0", "1"})
                n691 = local read "输入值_44"() -> (w161:enum16{"0", "1"})
                n692 = local read "输入值_45"() -> (w162:enum16{"0", "1"})
                n693 = local read "输入值_46"() -> (w163:enum16{"0", "1"})
                n694 = local read "输入值_47"() -> (w164:enum16{"0", "1"})
                n695 = local read "输入值_48"() -> (w165:enum16{"0", "1"})
                n696 = Build Array(w150, w151, w152, w153, w154, w155, w156, w157, w158, w159, w160, w161, w162, w163, w164, w165) -> (w148:enum16{"0", "1"}[])
                n697 = Build Array(w166, w167, w168, w169, w170, w171, w172, w173, w174, w175, w176, w177, w178, w179, w180, w181) -> (w149:bool[])
              }
              frame #3 {
                n698 = local read "单选_第49路"() -> (w200:bool)
                n699 = local read "单选_第50路"() -> (w201:bool)
                n700 = local read "单选_第51路"() -> (w202:bool)
                n701 = local read "单选_第52路"() -> (w203:bool)
                n702 = local read "单选_第53路"() -> (w204:bool)
                n703 = local read "单选_第54路"() -> (w205:bool)
                n704 = local read "单选_第55路"() -> (w206:bool)
                n705 = local read "单选_第56路"() -> (w207:bool)
                n706 = local read "单选_第57路"() -> (w208:bool)
                n707 = local read "单选_第58路"() -> (w209:bool)
                n708 = local read "单选_第59路"() -> (w210:bool)
                n709 = local read "单选_第60路"() -> (w211:bool)
                n710 = local read "单选_第61路"() -> (w212:bool)
                n711 = local read "单选_第62路"() -> (w213:bool)
                n712 = local read "单选_第63路"() -> (w214:bool)
                n713 = local read "单选_第64路"() -> (w215:bool)
                n714 = local read "输入值_49"() -> (w184:enum16{"0", "1"})
                n715 = local read "输入值_50"() -> (w185:enum16{"0", "1"})
                n716 = local read "输入值_51"() -> (w186:enum16{"0", "1"})
                n717 = local read "输入值_52"() -> (w187:enum16{"0", "1"})
                n718 = local read "输入值_53"() -> (w188:enum16{"0", "1"})
                n719 = local read "输入值_54"() -> (w189:enum16{"0", "1"})
                n720 = local read "输入值_55"() -> (w190:enum16{"0", "1"})
                n721 = local read "输入值_56"() -> (w191:enum16{"0", "1"})
                n722 = local read "输入值_57"() -> (w192:enum16{"0", "1"})
                n723 = local read "输入值_58"() -> (w193:enum16{"0", "1"})
                n724 = local read "输入值_59"() -> (w194:enum16{"0", "1"})
                n725 = local read "输入值_60"() -> (w195:enum16{"0", "1"})
                n726 = local read "输入值_61"() -> (w196:enum16{"0", "1"})
                n727 = local read "输入值_62"() -> (w197:enum16{"0", "1"})
                n728 = local read "输入值_63"() -> (w198:enum16{"0", "1"})
                n729 = local read "输入值_64"() -> (w199:enum16{"0", "1"})
                n730 = Build Array(w200, w201, w202, w203, w204, w205, w206, w207, w208, w209, w210, w211, w212, w213, w214, w215) -> (w183:bool[])
                n731 = Build Array(w184, w185, w186, w187, w188, w189, w190, w191, w192, w193, w194, w195, w196, w197, w198, w199) -> (w182:enum16{"0", "1"}[])
              }
              frame #4 {
                n732 = local read "单选_第71路"() -> (w240:bool)
                n733 = local read "单选_第79路"() -> (w248:bool)
                n734 = local read "单选_第65路"() -> (w234:bool)
                n735 = local read "单选_第66路"() -> (w235:bool)
                n736 = local read "单选_第67路"() -> (w236:bool)
                n737 = local read "单选_第68路"() -> (w237:bool)
                n738 = local read "单选_第69路"() -> (w238:bool)
                n739 = local read "单选_第70路"() -> (w239:bool)
                n740 = local read "单选_第72路"() -> (w241:bool)
                n741 = local read "单选_第73路"() -> (w242:bool)
                n742 = local read "单选_第74路"() -> (w243:bool)
                n743 = local read "单选_第75路"() -> (w244:bool)
                n744 = local read "单选_第76路"() -> (w245:bool)
                n745 = local read "单选_第77路"() -> (w246:bool)
                n746 = local read "单选_第78路"() -> (w247:bool)
                n747 = local read "单选_第80路"() -> (w249:bool)
                n748 = local read "输入值_65"() -> (w218:enum16{"0", "1"})
                n749 = local read "输入值_66"() -> (w219:enum16{"0", "1"})
                n750 = local read "输入值_67"() -> (w220:enum16{"0", "1"})
                n751 = local read "输入值_68"() -> (w221:enum16{"0", "1"})
                n752 = local read "输入值_69"() -> (w222:enum16{"0", "1"})
                n753 = local read "输入值_70"() -> (w223:enum16{"0", "1"})
                n754 = local read "输入值_71"() -> (w224:enum16{"0", "1"})
                n755 = local read "输入值_72"() -> (w225:enum16{"0", "1"})
                n756 = local read "输入值_73"() -> (w226:enum16{"0", "1"})
                n757 = local read "输入值_74"() -> (w227:enum16{"0", "1"})
                n758 = local read "输入值_75"() -> (w228:enum16{"0", "1"})
                n759 = local read "输入值_76"() -> (w229:enum16{"0", "1"})
                n760 = local read "输入值_77"() -> (w230:enum16{"0", "1"})
                n761 = local read "输入值_78"() -> (w231:enum16{"0", "1"})
                n762 = local read "输入值_79"() -> (w232:enum16{"0", "1"})
                n763 = local read "输入值_80"() -> (w233:enum16{"0", "1"})
                n764 = Build Array(w218, w219, w220, w221, w222, w223, w224, w225, w226, w227, w228, w229, w230, w231, w232, w233) -> (w216:enum16{"0", "1"}[])
                n765 = Build Array(w234, w235, w236, w237, w238, w239, w240, w241, w242, w243, w244, w245, w246, w247, w248, w249) -> (w217:bool[])
              }
            }
            n766 = local read "数组_选择?"() -> (w79:bool[][])
            n767 = local read "数组_输入值"() -> (w62:enum16{"0", "1"}[][])
            n768 = Replace Array Subset(array=w79, new element #1=w77, index (row) #1=0 ("索引 (行)"), new element #2=w75, index (row) #2=1 ("索引 (行)"), new element #3=w73, index (row) #3=2 ("索引 (行)"), new element #4=w71, index (row) #4=3 ("索引 (行)"), new element #5=w69, index (row) #5=4 ("索引 (行)")) -> (w68:bool[][])  [unwired: 5 in]
            n769 = local write "测试结论"("") -> ()
            n770 = local write "同步_A1"(w55) -> ()
            n771 = local write "同步_A2"(w55) -> ()
            n772 = Replace Array Subset(array=w62, new element #1=w61, index (row) #1=0 ("索引 (行)"), new element #2=w60, index (row) #2=1 ("索引 (行)"), new element #3=w59, index (row) #3=2 ("索引 (行)"), new element #4=w58, index (row) #4=3 ("索引 (行)"), new element #5=w57, index (row) #5=4 ("索引 (行)")) -> (w56:enum16{"0", "1"}[][])  [unwired: 5 in]
            n773 = local write "数组_输入值"(w56) -> ()
            n774 = local write "数组_选择?"(w68) -> ()
          }
          frame #1 {
            w250 = cluster{u32, u32}[] [{9868950, 9868950}]
            n775 = property on="light_1" class="Bool (严格)"("Colors [4]"=w250) -> ()  [unwired: 2 in, 2 out]
            n776 = property on="light_2" class="Bool (严格)"("Colors [4]"=w250) -> ()  [unwired: 2 in, 2 out]
            n777 = property on="light_3" class="Bool (严格)"("Colors [4]"=w250) -> ()  [unwired: 2 in, 2 out]
            n778 = property on="light_4" class="Bool (严格)"("Colors [4]"=w250) -> ()  [unwired: 2 in, 2 out]
            n779 = property on="light_5" class="Bool (严格)"("Colors [4]"=w250) -> ()  [unwired: 2 in, 2 out]
            n780 = property on="light_6" class="Bool (严格)"("Colors [4]"=w250) -> ()  [unwired: 2 in, 2 out]
            n781 = property on="light_7" class="Bool (严格)"("Colors [4]"=w250) -> ()  [unwired: 2 in, 2 out]
            n782 = property on="light_8" class="Bool (严格)"("Colors [4]"=w250) -> ()  [unwired: 2 in, 2 out]
            n783 = property on="light_9" class="Bool (严格)"("Colors [4]"=w250) -> ()  [unwired: 2 in, 2 out]
            n784 = property on="light_10" class="Bool (严格)"("Colors [4]"=w250) -> ()  [unwired: 2 in, 2 out]
            n785 = property on="light_11" class="Bool (严格)"("Colors [4]"=w250) -> ()  [unwired: 2 in, 2 out]
            n786 = property on="light_12" class="Bool (严格)"("Colors [4]"=w250) -> ()  [unwired: 2 in, 2 out]
            n787 = property on="light_13" class="Bool (严格)"("Colors [4]"=w250) -> ()  [unwired: 2 in, 2 out]
            n788 = property on="light_14" class="Bool (严格)"("Colors [4]"=w250) -> ()  [unwired: 2 in, 2 out]
            n789 = property on="light_15" class="Bool (严格)"("Colors [4]"=w250) -> ()  [unwired: 2 in, 2 out]
            n790 = property on="light_16" class="Bool (严格)"("Colors [4]"=w250) -> ()  [unwired: 2 in, 2 out]
            n791 = property on="light_17" class="Bool (严格)"("Colors [4]"=w250) -> ()  [unwired: 2 in, 2 out]
            n792 = property on="light_18" class="Bool (严格)"("Colors [4]"=w250) -> ()  [unwired: 2 in, 2 out]
            n793 = property on="light_19" class="Bool (严格)"("Colors [4]"=w250) -> ()  [unwired: 2 in, 2 out]
            n794 = property on="light_20" class="Bool (严格)"("Colors [4]"=w250) -> ()  [unwired: 2 in, 2 out]
            n795 = property on="light_21" class="Bool (严格)"("Colors [4]"=w250) -> ()  [unwired: 2 in, 2 out]
            n796 = property on="light_22" class="Bool (严格)"("Colors [4]"=w250) -> ()  [unwired: 2 in, 2 out]
            n797 = property on="light_23" class="Bool (严格)"("Colors [4]"=w250) -> ()  [unwired: 2 in, 2 out]
            n798 = property on="light_24" class="Bool (严格)"("Colors [4]"=w250) -> ()  [unwired: 2 in, 2 out]
            n799 = property on="light_25" class="Bool (严格)"("Colors [4]"=w250) -> ()  [unwired: 2 in, 2 out]
            n800 = property on="light_26" class="Bool (严格)"("Colors [4]"=w250) -> ()  [unwired: 2 in, 2 out]
            n801 = property on="light_27" class="Bool (严格)"("Colors [4]"=w250) -> ()  [unwired: 2 in, 2 out]
            n802 = property on="light_28" class="Bool (严格)"("Colors [4]"=w250) -> ()  [unwired: 2 in, 2 out]
            n803 = property on="light_29" class="Bool (严格)"("Colors [4]"=w250) -> ()  [unwired: 2 in, 2 out]
            n804 = property on="light_30" class="Bool (严格)"("Colors [4]"=w250) -> ()  [unwired: 2 in, 2 out]
            n805 = property on="light_31" class="Bool (严格)"("Colors [4]"=w250) -> ()  [unwired: 2 in, 2 out]
            n806 = property on="light_32" class="Bool (严格)"("Colors [4]"=w250) -> ()  [unwired: 2 in, 2 out]
            n807 = property on="light_33" class="Bool (严格)"("Colors [4]"=w250) -> ()  [unwired: 2 in, 2 out]
            n808 = property on="light_34" class="Bool (严格)"("Colors [4]"=w250) -> ()  [unwired: 2 in, 2 out]
            n809 = property on="light_35" class="Bool (严格)"("Colors [4]"=w250) -> ()  [unwired: 2 in, 2 out]
            n810 = property on="light_36" class="Bool (严格)"("Colors [4]"=w250) -> ()  [unwired: 2 in, 2 out]
            n811 = property on="light_37" class="Bool (严格)"("Colors [4]"=w250) -> ()  [unwired: 2 in, 2 out]
            n812 = property on="light_38" class="Bool (严格)"("Colors [4]"=w250) -> ()  [unwired: 2 in, 2 out]
            n813 = property on="light_39" class="Bool (严格)"("Colors [4]"=w250) -> ()  [unwired: 2 in, 2 out]
            n814 = property on="light_40" class="Bool (严格)"("Colors [4]"=w250) -> ()  [unwired: 2 in, 2 out]
            n815 = property on="light_41" class="Bool (严格)"("Colors [4]"=w250) -> ()  [unwired: 2 in, 2 out]
            n816 = property on="light_42" class="Bool (严格)"("Colors [4]"=w250) -> ()  [unwired: 2 in, 2 out]
            n817 = property on="light_43" class="Bool (严格)"("Colors [4]"=w250) -> ()  [unwired: 2 in, 2 out]
            n818 = property on="light_44" class="Bool (严格)"("Colors [4]"=w250) -> ()  [unwired: 2 in, 2 out]
            n819 = property on="light_45" class="Bool (严格)"("Colors [4]"=w250) -> ()  [unwired: 2 in, 2 out]
            n820 = property on="light_46" class="Bool (严格)"("Colors [4]"=w250) -> ()  [unwired: 2 in, 2 out]
            n821 = property on="light_47" class="Bool (严格)"("Colors [4]"=w250) -> ()  [unwired: 2 in, 2 out]
            n822 = property on="light_48" class="Bool (严格)"("Colors [4]"=w250) -> ()  [unwired: 2 in, 2 out]
            n823 = property on="light_49" class="Bool (严格)"("Colors [4]"=w250) -> ()  [unwired: 2 in, 2 out]
            n824 = property on="light_50" class="Bool (严格)"("Colors [4]"=w250) -> ()  [unwired: 2 in, 2 out]
            n825 = property on="light_51" class="Bool (严格)"("Colors [4]"=w250) -> ()  [unwired: 2 in, 2 out]
            n826 = property on="light_52" class="Bool (严格)"("Colors [4]"=w250) -> ()  [unwired: 2 in, 2 out]
            n827 = property on="light_53" class="Bool (严格)"("Colors [4]"=w250) -> ()  [unwired: 2 in, 2 out]
            n828 = property on="light_54" class="Bool (严格)"("Colors [4]"=w250) -> ()  [unwired: 2 in, 2 out]
            n829 = property on="light_55" class="Bool (严格)"("Colors [4]"=w250) -> ()  [unwired: 2 in, 2 out]
            n830 = property on="light_56" class="Bool (严格)"("Colors [4]"=w250) -> ()  [unwired: 2 in, 2 out]
            n831 = property on="light_57" class="Bool (严格)"("Colors [4]"=w250) -> ()  [unwired: 2 in, 2 out]
            n832 = property on="light_58" class="Bool (严格)"("Colors [4]"=w250) -> ()  [unwired: 2 in, 2 out]
            n833 = property on="light_59" class="Bool (严格)"("Colors [4]"=w250) -> ()  [unwired: 2 in, 2 out]
            n834 = property on="light_60" class="Bool (严格)"("Colors [4]"=w250) -> ()  [unwired: 2 in, 2 out]
            n835 = property on="light_61" class="Bool (严格)"("Colors [4]"=w250) -> ()  [unwired: 2 in, 2 out]
            n836 = property on="light_62" class="Bool (严格)"("Colors [4]"=w250) -> ()  [unwired: 2 in, 2 out]
            n837 = property on="light_63" class="Bool (严格)"("Colors [4]"=w250) -> ()  [unwired: 2 in, 2 out]
            n838 = property on="light_64" class="Bool (严格)"("Colors [4]"=w250) -> ()  [unwired: 2 in, 2 out]
            n839 = property on="light_65" class="Bool (严格)"("Colors [4]"=w250) -> ()  [unwired: 2 in, 2 out]
            n840 = property on="light_66" class="Bool (严格)"("Colors [4]"=w250) -> ()  [unwired: 2 in, 2 out]
            n841 = property on="light_67" class="Bool (严格)"("Colors [4]"=w250) -> ()  [unwired: 2 in, 2 out]
            n842 = property on="light_68" class="Bool (严格)"("Colors [4]"=w250) -> ()  [unwired: 2 in, 2 out]
            n843 = property on="light_69" class="Bool (严格)"("Colors [4]"=w250) -> ()  [unwired: 2 in, 2 out]
            n844 = property on="light_70" class="Bool (严格)"("Colors [4]"=w250) -> ()  [unwired: 2 in, 2 out]
            n845 = property on="light_71" class="Bool (严格)"("Colors [4]"=w250) -> ()  [unwired: 2 in, 2 out]
            n846 = property on="light_72" class="Bool (严格)"("Colors [4]"=w250) -> ()  [unwired: 2 in, 2 out]
            n847 = property on="light_73" class="Bool (严格)"("Colors [4]"=w250) -> ()  [unwired: 2 in, 2 out]
            n848 = property on="light_74" class="Bool (严格)"("Colors [4]"=w250) -> ()  [unwired: 2 in, 2 out]
            n849 = property on="light_75" class="Bool (严格)"("Colors [4]"=w250) -> ()  [unwired: 2 in, 2 out]
            n850 = property on="light_76" class="Bool (严格)"("Colors [4]"=w250) -> ()  [unwired: 2 in, 2 out]
            n851 = property on="light_77" class="Bool (严格)"("Colors [4]"=w250) -> ()  [unwired: 2 in, 2 out]
            n852 = property on="light_78" class="Bool (严格)"("Colors [4]"=w250) -> ()  [unwired: 2 in, 2 out]
            n853 = property on="light_79" class="Bool (严格)"("Colors [4]"=w250) -> ()  [unwired: 2 in, 2 out]
            n854 = property on="light_80" class="Bool (严格)"("Colors [4]"=w250) -> ()  [unwired: 2 in, 2 out]
            n855 = Initialize Array("", 16 ("维数大小"), 4 ("维数大小")) -> (w254:string[][])
            n856 = local write "D_IN_1"(w254) -> ()
            n857 = local write "D_IN_2"(w254) -> ()
            n858 = local write "D_IN_3"(w254) -> ()
            n859 = local write "D_IN_4"(w254) -> ()
            n860 = local write "D_IN_5"(w254) -> ()
          }
          frame #2 {
            n861 = local read "保持输出"() -> (w255:bool)
            n862 = case shown="假" w255 {
              frame False {
                n863 = property on="保持输出" class="Bool (严格)"("DisabledEnum"=T1."Disabled and Grayed Out" ("禁用")) -> ()  [unwired: 2 in, 2 out]
              }
              frame True {
                n864 = local read "数组_选择?"() -> (w257:bool[][])
                n865 = for {
                  tunnel: w257 -> [w261] mode=indexing
                  i -> [w259]
                  stop <- w258 stop-if-true
                  n866 = Or Array Elements(Boolean array=w261) -> (logical OR=w260:bool)
                  n867 = case shown="真" w260 {
                    tunnel: w259 -> [_ w263]
                    tunnel: [FALSE TRUE] -> w258
                    frame False {
                    }
                    frame True {
                      n868 = local write "同步_A1"(w263) -> ()
                      n869 = Increment(x=w263) -> (x+1=w267:i32)
                      n870 = Format Into String(format string="保持第%d组数据输出" ("格式字符串"), w267) -> (resulting string=w266:string)  [unwired: 2 in, 1 out]
                      n871 = call "显示对话框信息5"("Message"=w266) -> ("是"=w264:bool)  [unwired: 9 in, 1 out]
                      n872 = case shown="真" w264 {
                        tunnel: w263 -> [_ w269]
                        frame False {
                        }
                        frame True {
                          n873 = stacked-sequence {
                            tunnel: w269 -> [w270 _]
                            frame #0 {
                              n874 = for {
                                N: 5 -> [_]
                                tunnel: w270 -> [w273]
                                i -> [w272]
                                n875 = Not Equal?(x=w273, y=w272) -> (x != y?=w274:bool)
                                n876 = case shown="真" w274 {
                                tunnel: w272 -> [_ w278]
                                frame False {
                                }
                                frame True {
                                n877 = local read "数组_选择?"() -> (w280:bool[][])
                                n878 = Initialize Array(FALSE, 16 ("维数大小")) -> (w275:bool[])
                                n879 = Replace Array Subset(array=w280, new element=w275, index (row)=w278) -> (w279:bool[][])  [unwired: 1 in]
                                n880 = local write "数组_选择?"(w279) -> ()
                                }
                                }
                              }
                            }
                            frame #1 {
                              n881 = property on="btn_开始试验" class="Bool"("DisabledEnum"=T1."Disabled and Grayed Out" ("禁用")) -> ()  [unwired: 2 in, 2 out]
                            }
                          }
                        }
                      }
                      n882 = local write "保持输出"(w264) -> ()
                    }
                  }
                }
              }
            }
          }
          frame #3 {
            n883 = local read "数组_选择?"() -> (w283:bool[][])
            n884 = Or Array Elements(Boolean array=w283) -> (logical OR=w282:bool)
            n885 = case shown="真" w282 {
              frame False {
                n886 = call "显示对话框信息"("Message"="请选择数字量输入路数") -> ()  [unwired: 9 in, 2 out]
              }
              frame True {
                w286 = "DOStart" ("名称（未命名）")
                n887 = Obtain Notifier(name (unnamed)=w286, notification data type=w286) -> (notifier out=w285:refnum<notifier>)  [unwired: 2 in, 2 out]
                n888 = Send Notification(notification="DOutput" ("通知"), notifier=w285) -> ()  [unwired: 1 in, 2 out]
              }
            }
          }
        }
      }
      event "保持输出": Value Change {
        n889 = event-data() -> ()  [unwired: 1 in, 5 out]
        n890 = property on="btn_开始试验" class="Bool"("DisabledEnum"=T1."Enabled" ("禁用")) -> ()  [unwired: 2 in, 2 out]
      }
      event "btn_全选": Value Change {
        w289 = TRUE ("单选_第41路")
        n891 = event-data() -> ()  [unwired: 1 in, 5 out]
        n892 = local write "单选_第1路"(w289) -> ()
        n893 = local write "单选_第2路"(w289) -> ()
        n894 = local write "单选_第3路"(w289) -> ()
        n895 = local write "单选_第4路"(w289) -> ()
        n896 = local write "单选_第5路"(w289) -> ()
        n897 = local write "单选_第6路"(w289) -> ()
        n898 = local write "单选_第7路"(w289) -> ()
        n899 = local write "单选_第8路"(w289) -> ()
        n900 = local write "单选_第9路"(w289) -> ()
        n901 = local write "单选_第10路"(w289) -> ()
        n902 = local write "单选_第11路"(w289) -> ()
        n903 = local write "单选_第12路"(w289) -> ()
        n904 = local write "单选_第13路"(w289) -> ()
        n905 = local write "单选_第14路"(w289) -> ()
        n906 = local write "单选_第15路"(w289) -> ()
        n907 = local write "单选_第16路"(w289) -> ()
        n908 = local write "单选_第17路"(w289) -> ()
        n909 = local write "单选_第18路"(w289) -> ()
        n910 = local write "单选_第19路"(w289) -> ()
        n911 = local write "单选_第20路"(w289) -> ()
        n912 = local write "单选_第21路"(w289) -> ()
        n913 = local write "单选_第22路"(w289) -> ()
        n914 = local write "单选_第23路"(w289) -> ()
        n915 = local write "单选_第24路"(w289) -> ()
        n916 = local write "单选_第25路"(w289) -> ()
        n917 = local write "单选_第26路"(w289) -> ()
        n918 = local write "单选_第27路"(w289) -> ()
        n919 = local write "单选_第28路"(w289) -> ()
        n920 = local write "单选_第29路"(w289) -> ()
        n921 = local write "单选_第30路"(w289) -> ()
        n922 = local write "单选_第31路"(w289) -> ()
        n923 = local write "单选_第32路"(w289) -> ()
        n924 = local write "单选_第33路"(w289) -> ()
        n925 = local write "单选_第34路"(w289) -> ()
        n926 = local write "单选_第35路"(w289) -> ()
        n927 = local write "单选_第36路"(w289) -> ()
        n928 = local write "单选_第37路"(w289) -> ()
        n929 = local write "单选_第38路"(w289) -> ()
        n930 = local write "单选_第39路"(w289) -> ()
        n931 = local write "单选_第40路"(w289) -> ()
        n932 = local write "单选_第41路"(w289) -> ()
        n933 = local write "单选_第42路"(w289) -> ()
        n934 = local write "单选_第43路"(w289) -> ()
        n935 = local write "单选_第44路"(w289) -> ()
        n936 = local write "单选_第45路"(w289) -> ()
        n937 = local write "单选_第46路"(w289) -> ()
        n938 = local write "单选_第47路"(w289) -> ()
        n939 = local write "单选_第48路"(w289) -> ()
        n940 = local write "单选_第49路"(w289) -> ()
        n941 = local write "单选_第50路"(w289) -> ()
        n942 = local write "单选_第51路"(w289) -> ()
        n943 = local write "单选_第52路"(w289) -> ()
        n944 = local write "单选_第53路"(w289) -> ()
        n945 = local write "单选_第54路"(w289) -> ()
        n946 = local write "单选_第55路"(w289) -> ()
        n947 = local write "单选_第56路"(w289) -> ()
        n948 = local write "单选_第57路"(w289) -> ()
        n949 = local write "单选_第58路"(w289) -> ()
        n950 = local write "单选_第59路"(w289) -> ()
        n951 = local write "单选_第60路"(w289) -> ()
        n952 = local write "单选_第61路"(w289) -> ()
        n953 = local write "单选_第62路"(w289) -> ()
        n954 = local write "单选_第63路"(w289) -> ()
        n955 = local write "单选_第64路"(w289) -> ()
        n956 = local write "单选_第71路"(w289) -> ()
        n957 = local write "单选_第79路"(w289) -> ()
        n958 = local write "单选_第65路"(w289) -> ()
        n959 = local write "单选_第66路"(w289) -> ()
        n960 = local write "单选_第67路"(w289) -> ()
        n961 = local write "单选_第68路"(w289) -> ()
        n962 = local write "单选_第69路"(w289) -> ()
        n963 = local write "单选_第70路"(w289) -> ()
        n964 = local write "单选_第72路"(w289) -> ()
        n965 = local write "单选_第73路"(w289) -> ()
        n966 = local write "单选_第74路"(w289) -> ()
        n967 = local write "单选_第75路"(w289) -> ()
        n968 = local write "单选_第76路"(w289) -> ()
        n969 = local write "单选_第77路"(w289) -> ()
        n970 = local write "单选_第78路"(w289) -> ()
        n971 = local write "单选_第80路"(w289) -> ()
      }
      event "btn_反选": Value Change {
        n972 = event-data() -> ()  [unwired: 1 in, 5 out]
        n973 = local read "单选_第1路"() -> (w449:bool)
        n974 = local read "单选_第2路"() -> (w447:bool)
        n975 = local read "单选_第3路"() -> (w445:bool)
        n976 = local read "单选_第4路"() -> (w443:bool)
        n977 = local read "单选_第5路"() -> (w441:bool)
        n978 = local read "单选_第6路"() -> (w439:bool)
        n979 = local read "单选_第7路"() -> (w438:bool)
        n980 = local read "单选_第8路"() -> (w437:bool)
        n981 = local read "单选_第9路"() -> (w436:bool)
        n982 = local read "单选_第10路"() -> (w435:bool)
        n983 = local read "单选_第11路"() -> (w434:bool)
        n984 = local read "单选_第12路"() -> (w433:bool)
        n985 = local read "单选_第13路"() -> (w432:bool)
        n986 = local read "单选_第14路"() -> (w431:bool)
        n987 = local read "单选_第15路"() -> (w430:bool)
        n988 = local read "单选_第16路"() -> (w429:bool)
        n989 = local read "单选_第17路"() -> (w428:bool)
        n990 = local read "单选_第18路"() -> (w427:bool)
        n991 = local read "单选_第19路"() -> (w426:bool)
        n992 = local read "单选_第20路"() -> (w425:bool)
        n993 = local read "单选_第21路"() -> (w424:bool)
        n994 = local read "单选_第22路"() -> (w423:bool)
        n995 = local read "单选_第23路"() -> (w422:bool)
        n996 = local read "单选_第24路"() -> (w421:bool)
        n997 = local read "单选_第25路"() -> (w420:bool)
        n998 = local read "单选_第26路"() -> (w419:bool)
        n999 = local read "单选_第27路"() -> (w418:bool)
        n1000 = local read "单选_第28路"() -> (w417:bool)
        n1001 = local read "单选_第29路"() -> (w416:bool)
        n1002 = local read "单选_第30路"() -> (w415:bool)
        n1003 = local read "单选_第31路"() -> (w414:bool)
        n1004 = local read "单选_第32路"() -> (w413:bool)
        n1005 = local read "单选_第33路"() -> (w412:bool)
        n1006 = local read "单选_第34路"() -> (w411:bool)
        n1007 = local read "单选_第35路"() -> (w410:bool)
        n1008 = local read "单选_第36路"() -> (w409:bool)
        n1009 = local read "单选_第37路"() -> (w408:bool)
        n1010 = local read "单选_第38路"() -> (w407:bool)
        n1011 = local read "单选_第39路"() -> (w406:bool)
        n1012 = local read "单选_第40路"() -> (w405:bool)
        n1013 = Not(x=w449) -> (.not. x?=w448:bool)
        n1014 = Not(x=w447) -> (.not. x?=w446:bool)
        n1015 = Not(x=w445) -> (.not. x?=w444:bool)
        n1016 = Not(x=w443) -> (.not. x?=w442:bool)
        n1017 = Not(x=w441) -> (.not. x?=w440:bool)
        n1018 = Not(x=w439) -> (.not. x?=w404:bool)
        n1019 = Not(x=w438) -> (.not. x?=w403:bool)
        n1020 = Not(x=w437) -> (.not. x?=w402:bool)
        n1021 = Not(x=w436) -> (.not. x?=w401:bool)
        n1022 = Not(x=w435) -> (.not. x?=w400:bool)
        n1023 = Not(x=w434) -> (.not. x?=w399:bool)
        n1024 = Not(x=w433) -> (.not. x?=w398:bool)
        n1025 = Not(x=w432) -> (.not. x?=w397:bool)
        n1026 = Not(x=w431) -> (.not. x?=w396:bool)
        n1027 = Not(x=w430) -> (.not. x?=w395:bool)
        n1028 = Not(x=w429) -> (.not. x?=w394:bool)
        n1029 = Not(x=w428) -> (.not. x?=w393:bool)
        n1030 = Not(x=w427) -> (.not. x?=w392:bool)
        n1031 = Not(x=w426) -> (.not. x?=w391:bool)
        n1032 = Not(x=w425) -> (.not. x?=w390:bool)
        n1033 = Not(x=w424) -> (.not. x?=w389:bool)
        n1034 = Not(x=w423) -> (.not. x?=w388:bool)
        n1035 = Not(x=w422) -> (.not. x?=w387:bool)
        n1036 = Not(x=w421) -> (.not. x?=w386:bool)
        n1037 = Not(x=w420) -> (.not. x?=w385:bool)
        n1038 = Not(x=w419) -> (.not. x?=w384:bool)
        n1039 = Not(x=w418) -> (.not. x?=w383:bool)
        n1040 = Not(x=w417) -> (.not. x?=w382:bool)
        n1041 = Not(x=w416) -> (.not. x?=w381:bool)
        n1042 = Not(x=w415) -> (.not. x?=w380:bool)
        n1043 = Not(x=w414) -> (.not. x?=w379:bool)
        n1044 = Not(x=w413) -> (.not. x?=w378:bool)
        n1045 = Not(x=w412) -> (.not. x?=w377:bool)
        n1046 = Not(x=w411) -> (.not. x?=w376:bool)
        n1047 = Not(x=w410) -> (.not. x?=w375:bool)
        n1048 = Not(x=w409) -> (.not. x?=w374:bool)
        n1049 = Not(x=w408) -> (.not. x?=w373:bool)
        n1050 = Not(x=w407) -> (.not. x?=w372:bool)
        n1051 = Not(x=w406) -> (.not. x?=w371:bool)
        n1052 = Not(x=w405) -> (.not. x?=w370:bool)
        n1053 = local write "单选_第1路"(w448) -> ()
        n1054 = local write "单选_第2路"(w446) -> ()
        n1055 = local write "单选_第3路"(w444) -> ()
        n1056 = local write "单选_第4路"(w442) -> ()
        n1057 = local write "单选_第5路"(w440) -> ()
        n1058 = local write "单选_第6路"(w404) -> ()
        n1059 = local write "单选_第7路"(w403) -> ()
        n1060 = local write "单选_第8路"(w402) -> ()
        n1061 = local write "单选_第9路"(w401) -> ()
        n1062 = local write "单选_第10路"(w400) -> ()
        n1063 = local write "单选_第11路"(w399) -> ()
        n1064 = local write "单选_第12路"(w398) -> ()
        n1065 = local write "单选_第13路"(w397) -> ()
        n1066 = local write "单选_第14路"(w396) -> ()
        n1067 = local write "单选_第15路"(w395) -> ()
        n1068 = local write "单选_第16路"(w394) -> ()
        n1069 = local write "单选_第17路"(w393) -> ()
        n1070 = local write "单选_第18路"(w392) -> ()
        n1071 = local write "单选_第19路"(w391) -> ()
        n1072 = local write "单选_第20路"(w390) -> ()
        n1073 = local write "单选_第21路"(w389) -> ()
        n1074 = local write "单选_第22路"(w388) -> ()
        n1075 = local write "单选_第23路"(w387) -> ()
        n1076 = local write "单选_第24路"(w386) -> ()
        n1077 = local write "单选_第25路"(w385) -> ()
        n1078 = local write "单选_第26路"(w384) -> ()
        n1079 = local write "单选_第27路"(w383) -> ()
        n1080 = local write "单选_第28路"(w382) -> ()
        n1081 = local write "单选_第29路"(w381) -> ()
        n1082 = local write "单选_第30路"(w380) -> ()
        n1083 = local write "单选_第31路"(w379) -> ()
        n1084 = local write "单选_第32路"(w378) -> ()
        n1085 = local write "单选_第33路"(w377) -> ()
        n1086 = local write "单选_第34路"(w376) -> ()
        n1087 = local write "单选_第35路"(w375) -> ()
        n1088 = local write "单选_第36路"(w374) -> ()
        n1089 = local write "单选_第37路"(w373) -> ()
        n1090 = local write "单选_第38路"(w372) -> ()
        n1091 = local write "单选_第39路"(w371) -> ()
        n1092 = local write "单选_第40路"(w370) -> ()
        n1093 = local read "单选_第71路"() -> (w339:bool)
        n1094 = local read "单选_第79路"() -> (w331:bool)
        n1095 = local read "单选_第41路"() -> (w369:bool)
        n1096 = local read "单选_第42路"() -> (w368:bool)
        n1097 = local read "单选_第43路"() -> (w367:bool)
        n1098 = local read "单选_第44路"() -> (w366:bool)
        n1099 = local read "单选_第45路"() -> (w365:bool)
        n1100 = local read "单选_第46路"() -> (w364:bool)
        n1101 = local read "单选_第47路"() -> (w363:bool)
        n1102 = local read "单选_第48路"() -> (w362:bool)
        n1103 = local read "单选_第49路"() -> (w361:bool)
        n1104 = local read "单选_第50路"() -> (w360:bool)
        n1105 = local read "单选_第51路"() -> (w359:bool)
        n1106 = local read "单选_第52路"() -> (w358:bool)
        n1107 = local read "单选_第53路"() -> (w357:bool)
        n1108 = local read "单选_第54路"() -> (w356:bool)
        n1109 = local read "单选_第55路"() -> (w355:bool)
        n1110 = local read "单选_第56路"() -> (w354:bool)
        n1111 = local read "单选_第57路"() -> (w353:bool)
        n1112 = local read "单选_第58路"() -> (w352:bool)
        n1113 = local read "单选_第59路"() -> (w351:bool)
        n1114 = local read "单选_第60路"() -> (w350:bool)
        n1115 = local read "单选_第61路"() -> (w349:bool)
        n1116 = local read "单选_第62路"() -> (w348:bool)
        n1117 = local read "单选_第63路"() -> (w347:bool)
        n1118 = local read "单选_第64路"() -> (w346:bool)
        n1119 = local read "单选_第65路"() -> (w345:bool)
        n1120 = local read "单选_第66路"() -> (w344:bool)
        n1121 = local read "单选_第67路"() -> (w343:bool)
        n1122 = local read "单选_第68路"() -> (w342:bool)
        n1123 = local read "单选_第69路"() -> (w341:bool)
        n1124 = local read "单选_第70路"() -> (w340:bool)
        n1125 = local read "单选_第72路"() -> (w338:bool)
        n1126 = local read "单选_第73路"() -> (w337:bool)
        n1127 = local read "单选_第74路"() -> (w336:bool)
        n1128 = local read "单选_第75路"() -> (w335:bool)
        n1129 = local read "单选_第76路"() -> (w334:bool)
        n1130 = local read "单选_第77路"() -> (w333:bool)
        n1131 = local read "单选_第78路"() -> (w332:bool)
        n1132 = local read "单选_第80路"() -> (w330:bool)
        n1133 = Not(x=w369) -> (.not. x?=w329:bool)
        n1134 = Not(x=w368) -> (.not. x?=w328:bool)
        n1135 = Not(x=w367) -> (.not. x?=w327:bool)
        n1136 = Not(x=w366) -> (.not. x?=w326:bool)
        n1137 = Not(x=w365) -> (.not. x?=w325:bool)
        n1138 = Not(x=w364) -> (.not. x?=w324:bool)
        n1139 = Not(x=w363) -> (.not. x?=w323:bool)
        n1140 = Not(x=w362) -> (.not. x?=w322:bool)
        n1141 = Not(x=w361) -> (.not. x?=w321:bool)
        n1142 = Not(x=w360) -> (.not. x?=w320:bool)
        n1143 = Not(x=w359) -> (.not. x?=w319:bool)
        n1144 = Not(x=w358) -> (.not. x?=w318:bool)
        n1145 = Not(x=w357) -> (.not. x?=w317:bool)
        n1146 = Not(x=w356) -> (.not. x?=w316:bool)
        n1147 = Not(x=w355) -> (.not. x?=w315:bool)
        n1148 = Not(x=w354) -> (.not. x?=w314:bool)
        n1149 = Not(x=w353) -> (.not. x?=w313:bool)
        n1150 = Not(x=w352) -> (.not. x?=w312:bool)
        n1151 = Not(x=w351) -> (.not. x?=w311:bool)
        n1152 = Not(x=w350) -> (.not. x?=w310:bool)
        n1153 = Not(x=w349) -> (.not. x?=w309:bool)
        n1154 = Not(x=w348) -> (.not. x?=w308:bool)
        n1155 = Not(x=w347) -> (.not. x?=w307:bool)
        n1156 = Not(x=w346) -> (.not. x?=w306:bool)
        n1157 = Not(x=w345) -> (.not. x?=w305:bool)
        n1158 = Not(x=w344) -> (.not. x?=w304:bool)
        n1159 = Not(x=w343) -> (.not. x?=w303:bool)
        n1160 = Not(x=w342) -> (.not. x?=w302:bool)
        n1161 = Not(x=w341) -> (.not. x?=w301:bool)
        n1162 = Not(x=w340) -> (.not. x?=w300:bool)
        n1163 = Not(x=w339) -> (.not. x?=w299:bool)
        n1164 = Not(x=w338) -> (.not. x?=w298:bool)
        n1165 = Not(x=w337) -> (.not. x?=w297:bool)
        n1166 = Not(x=w336) -> (.not. x?=w296:bool)
        n1167 = Not(x=w335) -> (.not. x?=w295:bool)
        n1168 = Not(x=w334) -> (.not. x?=w294:bool)
        n1169 = Not(x=w333) -> (.not. x?=w293:bool)
        n1170 = Not(x=w332) -> (.not. x?=w292:bool)
        n1171 = Not(x=w331) -> (.not. x?=w291:bool)
        n1172 = Not(x=w330) -> (.not. x?=w290:bool)
        n1173 = local write "单选_第71路"(w299) -> ()
        n1174 = local write "单选_第79路"(w291) -> ()
        n1175 = local write "单选_第41路"(w329) -> ()
        n1176 = local write "单选_第42路"(w328) -> ()
        n1177 = local write "单选_第43路"(w327) -> ()
        n1178 = local write "单选_第44路"(w326) -> ()
        n1179 = local write "单选_第45路"(w325) -> ()
        n1180 = local write "单选_第46路"(w324) -> ()
        n1181 = local write "单选_第47路"(w323) -> ()
        n1182 = local write "单选_第48路"(w322) -> ()
        n1183 = local write "单选_第49路"(w321) -> ()
        n1184 = local write "单选_第50路"(w320) -> ()
        n1185 = local write "单选_第51路"(w319) -> ()
        n1186 = local write "单选_第52路"(w318) -> ()
        n1187 = local write "单选_第53路"(w317) -> ()
        n1188 = local write "单选_第54路"(w316) -> ()
        n1189 = local write "单选_第55路"(w315) -> ()
        n1190 = local write "单选_第56路"(w314) -> ()
        n1191 = local write "单选_第57路"(w313) -> ()
        n1192 = local write "单选_第58路"(w312) -> ()
        n1193 = local write "单选_第59路"(w311) -> ()
        n1194 = local write "单选_第60路"(w310) -> ()
        n1195 = local write "单选_第61路"(w309) -> ()
        n1196 = local write "单选_第62路"(w308) -> ()
        n1197 = local write "单选_第63路"(w307) -> ()
        n1198 = local write "单选_第64路"(w306) -> ()
        n1199 = local write "单选_第65路"(w305) -> ()
        n1200 = local write "单选_第66路"(w304) -> ()
        n1201 = local write "单选_第67路"(w303) -> ()
        n1202 = local write "单选_第68路"(w302) -> ()
        n1203 = local write "单选_第69路"(w301) -> ()
        n1204 = local write "单选_第70路"(w300) -> ()
        n1205 = local write "单选_第72路"(w298) -> ()
        n1206 = local write "单选_第73路"(w297) -> ()
        n1207 = local write "单选_第74路"(w296) -> ()
        n1208 = local write "单选_第75路"(w295) -> ()
        n1209 = local write "单选_第76路"(w294) -> ()
        n1210 = local write "单选_第77路"(w293) -> ()
        n1211 = local write "单选_第78路"(w292) -> ()
        n1212 = local write "单选_第80路"(w290) -> ()
      }
      event "btn_置1": Value Change {
        w450 = enum16{"0", "1"}."1" ("输入值_41")
        n1213 = event-data() -> ()  [unwired: 1 in, 5 out]
        n1214 = local write "输入值_1"(w450) -> ()
        n1215 = local write "输入值_2"(w450) -> ()
        n1216 = local write "输入值_3"(w450) -> ()
        n1217 = local write "输入值_4"(w450) -> ()
        n1218 = local write "输入值_5"(w450) -> ()
        n1219 = local write "输入值_6"(w450) -> ()
        n1220 = local write "输入值_7"(w450) -> ()
        n1221 = local write "输入值_8"(w450) -> ()
        n1222 = local write "输入值_9"(w450) -> ()
        n1223 = local write "输入值_10"(w450) -> ()
        n1224 = local write "输入值_11"(w450) -> ()
        n1225 = local write "输入值_12"(w450) -> ()
        n1226 = local write "输入值_13"(w450) -> ()
        n1227 = local write "输入值_14"(w450) -> ()
        n1228 = local write "输入值_15"(w450) -> ()
        n1229 = local write "输入值_16"(w450) -> ()
        n1230 = local write "输入值_17"(w450) -> ()
        n1231 = local write "输入值_18"(w450) -> ()
        n1232 = local write "输入值_19"(w450) -> ()
        n1233 = local write "输入值_20"(w450) -> ()
        n1234 = local write "输入值_21"(w450) -> ()
        n1235 = local write "输入值_22"(w450) -> ()
        n1236 = local write "输入值_23"(w450) -> ()
        n1237 = local write "输入值_24"(w450) -> ()
        n1238 = local write "输入值_25"(w450) -> ()
        n1239 = local write "输入值_26"(w450) -> ()
        n1240 = local write "输入值_27"(w450) -> ()
        n1241 = local write "输入值_28"(w450) -> ()
        n1242 = local write "输入值_29"(w450) -> ()
        n1243 = local write "输入值_30"(w450) -> ()
        n1244 = local write "输入值_31"(w450) -> ()
        n1245 = local write "输入值_32"(w450) -> ()
        n1246 = local write "输入值_33"(w450) -> ()
        n1247 = local write "输入值_34"(w450) -> ()
        n1248 = local write "输入值_35"(w450) -> ()
        n1249 = local write "输入值_36"(w450) -> ()
        n1250 = local write "输入值_37"(w450) -> ()
        n1251 = local write "输入值_38"(w450) -> ()
        n1252 = local write "输入值_39"(w450) -> ()
        n1253 = local write "输入值_40"(w450) -> ()
        n1254 = local write "输入值_41"(w450) -> ()
        n1255 = local write "输入值_42"(w450) -> ()
        n1256 = local write "输入值_43"(w450) -> ()
        n1257 = local write "输入值_44"(w450) -> ()
        n1258 = local write "输入值_45"(w450) -> ()
        n1259 = local write "输入值_46"(w450) -> ()
        n1260 = local write "输入值_47"(w450) -> ()
        n1261 = local write "输入值_48"(w450) -> ()
        n1262 = local write "输入值_49"(w450) -> ()
        n1263 = local write "输入值_50"(w450) -> ()
        n1264 = local write "输入值_51"(w450) -> ()
        n1265 = local write "输入值_52"(w450) -> ()
        n1266 = local write "输入值_53"(w450) -> ()
        n1267 = local write "输入值_54"(w450) -> ()
        n1268 = local write "输入值_55"(w450) -> ()
        n1269 = local write "输入值_56"(w450) -> ()
        n1270 = local write "输入值_57"(w450) -> ()
        n1271 = local write "输入值_58"(w450) -> ()
        n1272 = local write "输入值_59"(w450) -> ()
        n1273 = local write "输入值_60"(w450) -> ()
        n1274 = local write "输入值_61"(w450) -> ()
        n1275 = local write "输入值_62"(w450) -> ()
        n1276 = local write "输入值_63"(w450) -> ()
        n1277 = local write "输入值_64"(w450) -> ()
        n1278 = local write "输入值_65"(w450) -> ()
        n1279 = local write "输入值_66"(w450) -> ()
        n1280 = local write "输入值_67"(w450) -> ()
        n1281 = local write "输入值_68"(w450) -> ()
        n1282 = local write "输入值_69"(w450) -> ()
        n1283 = local write "输入值_70"(w450) -> ()
        n1284 = local write "输入值_71"(w450) -> ()
        n1285 = local write "输入值_72"(w450) -> ()
        n1286 = local write "输入值_73"(w450) -> ()
        n1287 = local write "输入值_74"(w450) -> ()
        n1288 = local write "输入值_75"(w450) -> ()
        n1289 = local write "输入值_76"(w450) -> ()
        n1290 = local write "输入值_77"(w450) -> ()
        n1291 = local write "输入值_78"(w450) -> ()
        n1292 = local write "输入值_79"(w450) -> ()
        n1293 = local write "输入值_80"(w450) -> ()
      }
      event "btn_置0": Value Change {
        w451 = enum16{"0", "1"}."0" ("输入值_41")
        n1294 = event-data() -> ()  [unwired: 1 in, 5 out]
        n1295 = local write "输入值_1"(w451) -> ()
        n1296 = local write "输入值_2"(w451) -> ()
        n1297 = local write "输入值_3"(w451) -> ()
        n1298 = local write "输入值_4"(w451) -> ()
        n1299 = local write "输入值_5"(w451) -> ()
        n1300 = local write "输入值_6"(w451) -> ()
        n1301 = local write "输入值_7"(w451) -> ()
        n1302 = local write "输入值_8"(w451) -> ()
        n1303 = local write "输入值_9"(w451) -> ()
        n1304 = local write "输入值_10"(w451) -> ()
        n1305 = local write "输入值_11"(w451) -> ()
        n1306 = local write "输入值_12"(w451) -> ()
        n1307 = local write "输入值_13"(w451) -> ()
        n1308 = local write "输入值_14"(w451) -> ()
        n1309 = local write "输入值_15"(w451) -> ()
        n1310 = local write "输入值_16"(w451) -> ()
        n1311 = local write "输入值_17"(w451) -> ()
        n1312 = local write "输入值_18"(w451) -> ()
        n1313 = local write "输入值_19"(w451) -> ()
        n1314 = local write "输入值_20"(w451) -> ()
        n1315 = local write "输入值_21"(w451) -> ()
        n1316 = local write "输入值_22"(w451) -> ()
        n1317 = local write "输入值_23"(w451) -> ()
        n1318 = local write "输入值_24"(w451) -> ()
        n1319 = local write "输入值_25"(w451) -> ()
        n1320 = local write "输入值_26"(w451) -> ()
        n1321 = local write "输入值_27"(w451) -> ()
        n1322 = local write "输入值_28"(w451) -> ()
        n1323 = local write "输入值_29"(w451) -> ()
        n1324 = local write "输入值_30"(w451) -> ()
        n1325 = local write "输入值_31"(w451) -> ()
        n1326 = local write "输入值_32"(w451) -> ()
        n1327 = local write "输入值_33"(w451) -> ()
        n1328 = local write "输入值_34"(w451) -> ()
        n1329 = local write "输入值_35"(w451) -> ()
        n1330 = local write "输入值_36"(w451) -> ()
        n1331 = local write "输入值_37"(w451) -> ()
        n1332 = local write "输入值_38"(w451) -> ()
        n1333 = local write "输入值_39"(w451) -> ()
        n1334 = local write "输入值_40"(w451) -> ()
        n1335 = local write "输入值_41"(w451) -> ()
        n1336 = local write "输入值_42"(w451) -> ()
        n1337 = local write "输入值_43"(w451) -> ()
        n1338 = local write "输入值_44"(w451) -> ()
        n1339 = local write "输入值_45"(w451) -> ()
        n1340 = local write "输入值_46"(w451) -> ()
        n1341 = local write "输入值_47"(w451) -> ()
        n1342 = local write "输入值_48"(w451) -> ()
        n1343 = local write "输入值_49"(w451) -> ()
        n1344 = local write "输入值_50"(w451) -> ()
        n1345 = local write "输入值_51"(w451) -> ()
        n1346 = local write "输入值_52"(w451) -> ()
        n1347 = local write "输入值_53"(w451) -> ()
        n1348 = local write "输入值_54"(w451) -> ()
        n1349 = local write "输入值_55"(w451) -> ()
        n1350 = local write "输入值_56"(w451) -> ()
        n1351 = local write "输入值_57"(w451) -> ()
        n1352 = local write "输入值_58"(w451) -> ()
        n1353 = local write "输入值_59"(w451) -> ()
        n1354 = local write "输入值_60"(w451) -> ()
        n1355 = local write "输入值_61"(w451) -> ()
        n1356 = local write "输入值_62"(w451) -> ()
        n1357 = local write "输入值_63"(w451) -> ()
        n1358 = local write "输入值_64"(w451) -> ()
        n1359 = local write "输入值_65"(w451) -> ()
        n1360 = local write "输入值_66"(w451) -> ()
        n1361 = local write "输入值_67"(w451) -> ()
        n1362 = local write "输入值_68"(w451) -> ()
        n1363 = local write "输入值_69"(w451) -> ()
        n1364 = local write "输入值_70"(w451) -> ()
        n1365 = local write "输入值_71"(w451) -> ()
        n1366 = local write "输入值_72"(w451) -> ()
        n1367 = local write "输入值_73"(w451) -> ()
        n1368 = local write "输入值_74"(w451) -> ()
        n1369 = local write "输入值_75"(w451) -> ()
        n1370 = local write "输入值_76"(w451) -> ()
        n1371 = local write "输入值_77"(w451) -> ()
        n1372 = local write "输入值_78"(w451) -> ()
        n1373 = local write "输入值_79"(w451) -> ()
        n1374 = local write "输入值_80"(w451) -> ()
      }
    }
  }
  n1375 = stacked-sequence {
    frame #0 {
      w452 = T1."Enabled" ("禁用")
      w453 = 0 ("同步_A1")
      w469 = T1."Disabled" ("禁用")
      n1376 = property on="测试结论" class="Str"("Text.TextColor"=u32 0) -> ()  [unwired: 2 in, 2 out]
      n1377 = local write "测试结论"("") -> ()
      n1378 = property on="D_IN_1" class="Tbl (严格)"("DisabledEnum"=w469) -> ()  [unwired: 2 in, 2 out]
      n1379 = property on="D_IN_2" class="Tbl (严格)"("DisabledEnum"=w469) -> ()  [unwired: 2 in, 2 out]
      n1380 = property on="D_IN_3" class="Tbl (严格)"("DisabledEnum"=w469) -> ()  [unwired: 2 in, 2 out]
      n1381 = property on="D_IN_4" class="Tbl (严格)"("DisabledEnum"=w469) -> ()  [unwired: 2 in, 2 out]
      n1382 = property on="D_IN_5" class="Tbl (严格)"("DisabledEnum"=w469) -> ()  [unwired: 2 in, 2 out]
      n1383 = property on="保持输出" class="Bool (严格)"("DisabledEnum"=w452) -> ()  [unwired: 2 in, 2 out]
      n1384 = property on="btn_开始试验" class="Bool"("DisabledEnum"=w452) -> ()  [unwired: 2 in, 2 out]
      n1385 = for {
        N: 16 -> [_]
        i -> [w473]
        n1386 = for {
          N: 4 -> [_]
          tunnel: w473 -> [w477]
          i -> [w478]
          w475 = u32 24 ("活动单元格:单元格大小:高度")
          n1387 = Bundle(w477, w478) -> (w476:cluster{i32, i32})  [unwired: 1 in]
          n1388 = property on="D_IN_1" class="Tbl (严格)"("Active Cell"=w476) -> (error out=w479:errorcluster)  [unwired: 2 in, 1 out]
          n1389 = property on="D_IN_2" class="Tbl (严格)"("Active Cell"=w476) -> ()  [unwired: 2 in, 2 out]
          n1390 = property on="D_IN_3" class="Tbl (严格)"("Active Cell"=w476) -> ()  [unwired: 2 in, 2 out]
          n1391 = property on="D_IN_4" class="Tbl (严格)"("Active Cell"=w476) -> ()  [unwired: 2 in, 2 out]
          n1392 = property on="D_IN_5" class="Tbl (严格)"("Active Cell"=w476) -> ()  [unwired: 2 in, 2 out]
          n1393 = property on="D_IN_1" class="Tbl (严格)"(error in=w479, "Height"=w475) -> ()  [unwired: 1 in, 2 out]
          n1394 = property on="D_IN_2" class="Tbl (严格)"("Height"=w475) -> ()  [unwired: 2 in, 2 out]
          n1395 = property on="D_IN_3" class="Tbl (严格)"("Height"=w475) -> ()  [unwired: 2 in, 2 out]
          n1396 = property on="D_IN_4" class="Tbl (严格)"("Height"=w475) -> ()  [unwired: 2 in, 2 out]
          n1397 = property on="D_IN_5" class="Tbl (严格)"("Height"=w475) -> ()  [unwired: 2 in, 2 out]
        }
        n1398 = Wait Until Next ms Multiple(millisecond multiple=u32 10 ("毫秒倍数")) -> ()  [unwired: 1 out]
      }
      n1399 = Initialize Array(FALSE, 5 ("维数大小"), 16 ("维数大小")) -> (w461:bool[][])
      n1400 = Initialize Array(enum16{"0", "1"}."0" ("输入值_32"), 5 ("维数大小"), 16 ("维数大小")) -> (w455:enum16{"0", "1"}[][])
      n1401 = Initialize Array("", 16 ("维数大小"), 4 ("维数大小")) -> (w463:string[][])
      n1402 = local write "关闭？"(FALSE) -> ()
      n1403 = local write "CAN端口"(u16 1 ("CAN端口")) -> ()
      n1404 = local write "数组_选择?"(w461) -> ()
      n1405 = local write "数组_输入值"(w455) -> ()
      n1406 = local write "D_IN_1"(w463) -> ()
      n1407 = local write "D_IN_2"(w463) -> ()
      n1408 = local write "D_IN_3"(w463) -> ()
      n1409 = local write "D_IN_4"(w463) -> ()
      n1410 = local write "D_IN_5"(w463) -> ()
      n1411 = local write "同步_A1"(w453) -> ()
      n1412 = local write "同步_A2"(w453) -> ()
    }
  }
  n1413 = Obtain Notifier(name (unnamed)=w8, notification data type=w8) -> (notifier out=w10:refnum<notifier>, error out=w9:errorcluster)  [unwired: 2 in, 1 out]
  n1414 = while {
    tunnel: w10 -> [w483]
    tunnel: w9 -> [w482]
    tunnel: [w481] -> w7
    tunnel: [w480] -> w6
    stop <- w484 stop-if-true
    n1415 = Wait Until Next ms Multiple(millisecond multiple=u32 20 ("毫秒倍数")) -> ()  [unwired: 1 out]
    n1416 = Wait on Notification(notifier=w483, timeout in ms (-1)=20 ("超时毫秒(-1)"), error in (no error)=w482) -> (notifier out=w481:refnum<notifier>, notification=w489:string, error out=w480:errorcluster)  [unwired: 1 in, 1 out]
    n1417 = Equal?(x=w489, y="DOutput" ("通知")) -> (x = y?=w487:bool)
    n1418 = case shown="真" w487 {
      frame False {
      }
      frame True {
        n1419 = while {
          stop <- w491 stop-if-true
          n1420 = local read "保持输出"() -> (w490:bool)
          n1421 = case shown="真" w490 {
            selector: w490 -> [_ w525]
            tunnel: [w496 w526] -> w493
            tunnel: [w495 w524] -> w492
            frame False {
              n1422 = stacked-sequence {
                tunnel: [_ w520] -> w495
                tunnel: [w498 _] -> w496
                frame #0 {
                  n1423 = local read "同步_A2"() -> (w500:i32)
                  n1424 = local read "同步_A1"() -> (w497:i32)
                  n1425 = Equal?(x=w497, y=w500) -> (x = y?=w499:bool)
                  n1426 = case shown="真" w499 {
                    tunnel: [FALSE w502] -> w498
                    frame False {
                    }
                    frame True {
                      n1427 = stacked-sequence {
                        tunnel: [_ w512 _] -> w502
                        frame #0 {
                          w504 = "DOCheckStart" ("名称（未命名）")
                          n1428 = Obtain Notifier(name (unnamed)=w504, notification data type=w504) -> (notifier out=w505:refnum<notifier>)  [unwired: 2 in, 2 out]
                          n1429 = Send Notification(notification="DOCheck" ("通知"), notifier=w505) -> ()  [unwired: 1 in, 2 out]
                        }
                        frame #1 {
                          # "32+16+PWM+16(I/O)\n4X3=12   每次一组"
                          # "以太网发送修改数字量输出参数命令"
                          n1430 = local read "数组_输入值"() -> (w514:enum16{"0", "1"}[][])
                          n1431 = local read "同步_A1"() -> (w510:i32)
                          n1432 = call "数值转换为U16.vi"("数值数组输入"=w514) -> ("U16输出"=w511:u16[])  [unwired: 10 in]
                          n1433 = Multiply(x=w510, y=3) -> (x*y=w508:i32)
                          n1434 = Array Subset(array=w511, index=w508, length=3 ("长度")) -> (w506:u16[])
                          n1435 = call "UDP发送.vi"("发送数据"=w506, "数据区字长"=u16 3, "报文类型"=u16 1285, "发送方标识"=u16 5397) -> ("Error"=w513:cluster{"错误？":bool, "数值":i32, "字符串":string})  [unwired: 6 in]
                          n1436 = Unbundle By Name(w513) -> ("错误？"=w512:bool)
                        }
                        frame #2 {
                          n1437 = local read "同步_A1"() -> (w518:i32)
                          n1438 = Increment(x=w518) -> (x+1=w519:i32)
                          n1439 = local write "同步_A1"(w519) -> ()
                        }
                      }
                    }
                  }
                }
                frame #1 {
                  n1440 = local read "同步_A1"() -> (w521:i32)
                  n1441 = Equal?(x=w521, y=5) -> (x = y?=w520:bool)
                  n1442 = case shown="真" w520 {
                    frame False {
                    }
                    frame True {
                      n1443 = property on="保持输出" class="Bool (严格)"("DisabledEnum"=T1."Enabled" ("禁用")) -> ()  [unwired: 2 in, 2 out]
                    }
                  }
                }
              }
            }
            frame True {
              n1444 = Not(x=w525) -> (.not. x?=w524:bool)
              n1445 = stacked-sequence {
                tunnel: [_ w536] -> w526
                frame #0 {
                  w528 = "DOCheckStart" ("名称（未命名）")
                  n1446 = Obtain Notifier(name (unnamed)=w528, notification data type=w528) -> (notifier out=w529:refnum<notifier>)  [unwired: 2 in, 2 out]
                  n1447 = Send Notification(notification="DOCheck" ("通知"), notifier=w529) -> ()  [unwired: 1 in, 2 out]
                }
                frame #1 {
                  # "32+16+PWM+16(I/O)\n4X3=12，每次一组"
                  # "以太网发送修改数字量输出参数命令"
                  n1448 = local read "数组_输入值"() -> (w538:enum16{"0", "1"}[][])
                  n1449 = local read "同步_A1"() -> (w534:i32)
                  n1450 = call "数值转换为U16.vi"("数值数组输入"=w538) -> ("U16输出"=w535:u16[])  [unwired: 10 in]
                  n1451 = Multiply(x=w534, y=3) -> (x*y=w532:i32)
                  n1452 = Array Subset(array=w535, index=w532, length=3 ("长度")) -> (w530:u16[])
                  n1453 = call "UDP发送.vi"("发送数据"=w530, "数据区字长"=u16 3, "报文类型"=u16 1285, "发送方标识"=u16 5397) -> ("Error"=w537:cluster{"错误？":bool, "数值":i32, "字符串":string})  [unwired: 6 in]
                  n1454 = Unbundle By Name(w537) -> ("错误？"=w536:bool)
                }
              }
            }
          }
          n1455 = Wait Until Next ms Multiple(millisecond multiple=u32 25 ("毫秒倍数")) -> ()  [unwired: 1 out]
          n1456 = Or(x=w493, y=w492) -> (x .or. y?=w491:bool)
        }
      }
    }
    n1457 = local read "关闭？"() -> (w484:bool)
  }
  n1458 = Release Notifier(notifier=w7, error in (no error)=w6) -> ()  [unwired: 1 in, 3 out]
  n1459 = disable-structure shown="禁用" {
    frame Disabled {
      n1460 = for {
        N: 40 -> [_]
        i -> [w547]
        n1461 = Wait Until Next ms Multiple(millisecond multiple=u32 10 ("毫秒倍数")) -> ()  [unwired: 1 out]
        n1462 = Bundle(w547, "y"=-1) -> (w546:cluster{i32, "y":i32})  [unwired: 1 in]
        n1463 = property on="D_IN_1" class="Tbl (严格)"("Active Cell"=w546) -> (error out=w545:errorcluster)  [unwired: 2 in, 1 out]
        n1464 = property on="D_IN_1" class="Tbl (严格)"(error in=w545, "Cell BG Color"=u32 12369084) -> ()  [unwired: 1 in, 2 out]
      }
    }
    frame Enabled {
    }
  }
  n1465 = disable-structure shown="禁用" {
    frame Disabled {
      n1466 = for {
        N: 40 -> [_]
        i -> [w551]
        n1467 = for {
          N: 4 -> [_]
          tunnel: w551 -> [w559]
          i -> [w556]
          n1468 = Bundle(w559, w556) -> (w555:cluster{i32, i32})  [unwired: 1 in]
          n1469 = Quotient & Remainder(x=w559, y=2) -> (x-y*floor(x/y)=w557:i32)  [unwired: 1 out]
          n1470 = property on="D_IN_1" class="Tbl (严格)"("Active Cell"=w555) -> (error out=w553:errorcluster)  [unwired: 2 in, 1 out]
          n1471 = Equal To 0?(x=w557) -> (x = 0?=w560:bool)
          n1472 = case shown="真" w560 {
            tunnel: [u32 16448250 u32 15723488] -> w554
            frame False {
            }
            frame True {
            }
          }
          n1473 = property on="D_IN_1" class="Tbl (严格)"(error in=w553, "Cell BG Color"=w554) -> ()  [unwired: 1 in, 2 out]
        }
        n1474 = Wait Until Next ms Multiple(millisecond multiple=u32 10 ("毫秒倍数")) -> ()  [unwired: 1 out]
      }
    }
    frame Enabled {
    }
  }
  n1475 = Obtain Notifier(name (unnamed)=w5, notification data type=w5) -> (notifier out=w4:refnum<notifier>, error out=w3:errorcluster)  [unwired: 2 in, 1 out]
  n1476 = while {
    tunnel: w4 -> [w566]
    tunnel: w3 -> [w565]
    tunnel: [w564] -> w2
    tunnel: [w563] -> w1
    stop <- w568 stop-if-true
    n1477 = Wait Until Next ms Multiple(millisecond multiple=u32 20 ("毫秒倍数")) -> ()  [unwired: 1 out]
    n1478 = Wait on Notification(notifier=w566, timeout in ms (-1)=20 ("超时毫秒(-1)"), error in (no error)=w565) -> (notifier out=w564:refnum<notifier>, notification=w569:string, error out=w563:errorcluster)  [unwired: 1 in, 1 out]
    n1479 = Equal?(x=w569, y="DOCheck" ("通知")) -> (x = y?=w567:bool)
    n1480 = case shown="真" w567 {
      frame False {
      }
      frame True {
        n1481 = stacked-sequence {
          frame #0 {
            w575 = u16 0
            w579 = u16 5397
            # "异常"
            # "正常"
            n1482 = Build Array(w579, u16 1285, w575) -> (w581:u16[])
            n1483 = Build Array(w579, u16 34181, u16 0 ("元素")) -> (w578:u16[])
            n1484 = Add(x=w575, y=u16 4) -> (x+y=w573:u16)
            n1485 = call "UDP接收.vi"("匹配帧信息_异常"=w578, "长度"=w573, "匹配帧信息_正常"=w581) -> ("异常_找到?"=w584:bool, "接收超时?"=w583:bool, "正常_找到?"=w576:bool)  [unwired: 5 in, 1 out]
            n1486 = case shown="真" w576 {
              frame False {
                n1487 = disable-structure shown="禁用" {
                  frame Disabled {
                    n1488 = call "显示对话框信息4"("Message"="以太网接收数据错误") -> ()  [unwired: 9 in, 2 out]
                  }
                  frame Enabled {
                  }
                }
              }
              frame True {
                n1489 = local read "保持输出"() -> (w595:bool)
                n1490 = local read "数组_输入值"() -> (w599:enum16{"0", "1"}[][])
                n1491 = local read "数组_选择?"() -> (w600:bool[][])
                n1492 = local read "CAN端口"() -> (w601:u16)
                n1493 = case shown="假" w595 {
                  tunnel: [w603 w604] -> w598
                  frame False {
                    n1494 = local read "同步_A2"() -> (w603:i32)
                  }
                  frame True {
                    n1495 = local read "同步_A1"() -> (w604:i32)
                  }
                }
                n1496 = Index Array(array=w600, index (row)=w598) -> (element=w596:bool[])  [unwired: 1 in]
                n1497 = To Unsigned Byte Integer(number=w598) -> (unsigned 8bit integer=w594:u8)
                n1498 = Index Array(array=w599, index (row)=w598) -> (element=w602:enum16{"0", "1"}[])  [unwired: 1 in]
                n1499 = Or Array Elements(Boolean array=w596) -> (logical OR=w597:bool)
                n1500 = case shown="真" w597 {
                  tunnel: w602 -> [_ w606]
                  tunnel: w594 -> [_ w610]
                  tunnel: w601 -> [_ w609]
                  tunnel: w598 -> [_ w608]
                  tunnel: w596 -> [_ w607]
                  frame False {
                  }
                  frame True {
                    n1501 = call "16路数字量输出.vi"("第几组数据"=w610, "CAN端口"=w609) -> ("成功?"=w605:bool)  [unwired: 9 in]
                    n1502 = case shown="真" w605 {
                      tunnel: w608 -> [_ w633]
                      tunnel: w607 -> [_ w625]
                      tunnel: w606 -> [_ w623]
                      frame False {
                      }
                      frame True {
                        n1503 = call "DAQNavi Assistant2"() -> ("dataOut(U8Array)"=w621:u8[])  [unwired: 2 in, 17 out]
                        n1504 = Index Array(array=w621, index #1=0 ("索引"), index #2=1 ("索引")) -> (element #1=w618:u8, element #2=w617:u8)
                        n1505 = local read "保持输出"() -> (w611:bool)
                        n1506 = Number To Boolean Array(number=w618) -> (Boolean array=w614:bool[])
                        n1507 = Number To Boolean Array(number=w617) -> (Boolean array=w613:bool[])
                        n1508 = Build Array (concatenate)(w614, w613) -> (w616:bool[])
                        n1509 = Boolean To (0,1)(Boolean=w616) -> (0, 1=w615:i16[])
                        n1510 = case shown="真" w611 {
                          tunnel: [w634 w635] -> w612
                          frame False {
                            n1511 = local read "同步_A2"() -> (w634:i32)
                          }
                          frame True {
                            n1512 = local read "同步_A1"() -> (w635:i32)
                          }
                        }
                        n1513 = for {
                          tunnel: w615 -> [w641] mode=indexing
                          tunnel: w623 -> [w640] mode=indexing
                          tunnel: w625 -> [w639] mode=indexing
                          tunnel: [w636] -> w626 mode=indexing
                          tunnel: [w637] -> w627 mode=indexing
                          tunnel: [w638] -> w622 mode=indexing
                          n1514 = case shown="真" w639 {
                            tunnel: w641 -> [_ w649]
                            tunnel: w640 -> [_ w651]
                            tunnel: [cluster{u32, u32}[] [{12369084, 12369084}] ("结果") w645] -> w636
                            tunnel: ["" w647] -> w637
                            tunnel: [TRUE w646] -> w638
                            frame False {
                            }
                            frame True {
                              n1515 = To Word Integer(number=w651) -> (16bit integer=w650:i16)
                              n1516 = Equal To 0?(x=w649) -> (x = 0?=w648:bool)
                              n1517 = Equal?(x=w649, y=w650) -> (x = y?=w646:bool)
                              n1518 = case shown="假" w646 {
                                tunnel: [cluster{u32, u32}[] [{16711680, 16711680}] ("结果") cluster{u32, u32}[] [{6618880, 6618880}] ("结果")] -> w645
                                frame False {
                                }
                                frame True {
                                }
                              }
                              n1519 = case shown="真" w648 {
                                tunnel: ["1" "0"] -> w647
                                frame False {
                                }
                                frame True {
                                }
                              }
                            }
                          }
                        }
                        n1520 = local read "测试结论"() -> (w631:string)
                        n1521 = And Array Elements(Boolean array=w622) -> (logical AND=w624:bool)
                        n1522 = case shown="真" w624 {
                          tunnel: ["被测板卡所选择的数字量输出%d组测试故障，具体见上面试验结论！" "被测板卡所选择的数字量输出%d组测试正常！"] -> w629
                          frame False {
                          }
                          frame True {
                          }
                        }
                        n1523 = Format Into String(format string=w629, w612) -> (resulting string=w632:string)  [unwired: 2 in, 1 out]
                        n1524 = Concatenate Strings(w631, w632, "\r") -> (w628:string)
                        n1525 = local write "测试结论"(w628) -> ()
                        n1526 = case shown="4" w633 {
                          tunnel: w626 -> [w660 w713 w750 w787 w824]
                          tunnel: w627 -> [w656 w694 w731 w767 w804]
                          frame 0, Default {
                            n1527 = local read "D_IN_1"() -> (w659:string[][])
                            n1528 = Replace Array Subset(array=w659, new element=w656, index (col)=2 ("禁用的索引 (列)")) -> (w657:string[][])  [unwired: 1 in]
                            n1529 = Index Array(array=w660, index (row) #1=0 ("索引"), index (row) #2=1 ("索引"), index (row) #3=2 ("索引"), index (row) #4=3 ("索引"), index (row) #5=4 ("索引"), index (row) #6=5 ("索引"), index (row) #7=6 ("索引"), index (row) #8=7 ("索引"), index (row) #9=8 ("索引"), index (row) #10=9 ("索引"), index (row) #11=10 ("索引"), index (row) #12=11 ("索引"), index (row) #13=12 ("索引"), index (row) #14=13 ("索引"), index (row) #15=14 ("索引"), index (row) #16=15 ("索引")) -> (element #1=w676:cluster{u32, u32}[], element #2=w675:cluster{u32, u32}[], element #3=w674:cluster{u32, u32}[], element #4=w673:cluster{u32, u32}[], element #5=w672:cluster{u32, u32}[], element #6=w661:cluster{u32, u32}[], element #7=w662:cluster{u32, u32}[], element #8=w663:cluster{u32, u32}[], element #9=w664:cluster{u32, u32}[], element #10=w665:cluster{u32, u32}[], element #11=w666:cluster{u32, u32}[], element #12=w667:cluster{u32, u32}[], element #13=w668:cluster{u32, u32}[], element #14=w669:cluster{u32, u32}[], element #15=w670:cluster{u32, u32}[], element #16=w671:cluster{u32, u32}[])  [unwired: 16 in]
                            n1530 = local write "D_IN_1"(w657) -> ()
                            n1531 = property on="light_1" class="Bool (严格)"("Colors [4]"=w676) -> ()  [unwired: 2 in, 2 out]
                            n1532 = property on="light_2" class="Bool (严格)"("Colors [4]"=w675) -> ()  [unwired: 2 in, 2 out]
                            n1533 = property on="light_3" class="Bool (严格)"("Colors [4]"=w674) -> ()  [unwired: 2 in, 2 out]
                            n1534 = property on="light_4" class="Bool (严格)"("Colors [4]"=w673) -> ()  [unwired: 2 in, 2 out]
                            n1535 = property on="light_5" class="Bool (严格)"("Colors [4]"=w672) -> ()  [unwired: 2 in, 2 out]
                            n1536 = property on="light_6" class="Bool (严格)"("Colors [4]"=w661) -> ()  [unwired: 2 in, 2 out]
                            n1537 = property on="light_7" class="Bool (严格)"("Colors [4]"=w662) -> ()  [unwired: 2 in, 2 out]
                            n1538 = property on="light_8" class="Bool (严格)"("Colors [4]"=w663) -> ()  [unwired: 2 in, 2 out]
                            n1539 = property on="light_9" class="Bool (严格)"("Colors [4]"=w664) -> ()  [unwired: 2 in, 2 out]
                            n1540 = property on="light_10" class="Bool (严格)"("Colors [4]"=w665) -> ()  [unwired: 2 in, 2 out]
                            n1541 = property on="light_11" class="Bool (严格)"("Colors [4]"=w666) -> ()  [unwired: 2 in, 2 out]
                            n1542 = property on="light_12" class="Bool (严格)"("Colors [4]"=w667) -> ()  [unwired: 2 in, 2 out]
                            n1543 = property on="light_13" class="Bool (严格)"("Colors [4]"=w668) -> ()  [unwired: 2 in, 2 out]
                            n1544 = property on="light_14" class="Bool (严格)"("Colors [4]"=w669) -> ()  [unwired: 2 in, 2 out]
                            n1545 = property on="light_15" class="Bool (严格)"("Colors [4]"=w670) -> ()  [unwired: 2 in, 2 out]
                            n1546 = property on="light_16" class="Bool (严格)"("Colors [4]"=w671) -> ()  [unwired: 2 in, 2 out]
                          }
                          frame 2 {
                            n1547 = local read "D_IN_3"() -> (w695:string[][])
                            n1548 = Replace Array Subset(array=w695, new element=w694, index (col)=2 ("索引 (列)")) -> (w693:string[][])  [unwired: 1 in]
                            n1549 = Index Array(array=w713, index (row) #1=0 ("索引"), index (row) #2=1 ("索引"), index (row) #3=2 ("索引"), index (row) #4=3 ("索引"), index (row) #5=4 ("索引"), index (row) #6=5 ("索引"), index (row) #7=6 ("索引"), index (row) #8=7 ("索引"), index (row) #9=8 ("索引"), index (row) #10=9 ("索引"), index (row) #11=10 ("索引"), index (row) #12=11 ("索引"), index (row) #13=12 ("索引"), index (row) #14=13 ("索引"), index (row) #15=14 ("索引"), index (row) #16=15 ("索引")) -> (element #1=w712:cluster{u32, u32}[], element #2=w711:cluster{u32, u32}[], element #3=w710:cluster{u32, u32}[], element #4=w709:cluster{u32, u32}[], element #5=w708:cluster{u32, u32}[], element #6=w707:cluster{u32, u32}[], element #7=w706:cluster{u32, u32}[], element #8=w705:cluster{u32, u32}[], element #9=w704:cluster{u32, u32}[], element #10=w703:cluster{u32, u32}[], element #11=w702:cluster{u32, u32}[], element #12=w701:cluster{u32, u32}[], element #13=w700:cluster{u32, u32}[], element #14=w699:cluster{u32, u32}[], element #15=w698:cluster{u32, u32}[], element #16=w697:cluster{u32, u32}[])  [unwired: 16 in]
                            n1550 = local write "D_IN_3"(w693) -> ()
                            n1551 = property on="light_33" class="Bool (严格)"("Colors [4]"=w712) -> ()  [unwired: 2 in, 2 out]
                            n1552 = property on="light_34" class="Bool (严格)"("Colors [4]"=w711) -> ()  [unwired: 2 in, 2 out]
                            n1553 = property on="light_35" class="Bool (严格)"("Colors [4]"=w710) -> ()  [unwired: 2 in, 2 out]
                            n1554 = property on="light_36" class="Bool (严格)"("Colors [4]"=w709) -> ()  [unwired: 2 in, 2 out]
                            n1555 = property on="light_37" class="Bool (严格)"("Colors [4]"=w708) -> ()  [unwired: 2 in, 2 out]
                            n1556 = property on="light_38" class="Bool (严格)"("Colors [4]"=w707) -> ()  [unwired: 2 in, 2 out]
                            n1557 = property on="light_39" class="Bool (严格)"("Colors [4]"=w706) -> ()  [unwired: 2 in, 2 out]
                            n1558 = property on="light_40" class="Bool (严格)"("Colors [4]"=w705) -> ()  [unwired: 2 in, 2 out]
                            n1559 = property on="light_41" class="Bool (严格)"("Colors [4]"=w704) -> ()  [unwired: 2 in, 2 out]
                            n1560 = property on="light_42" class="Bool (严格)"("Colors [4]"=w703) -> ()  [unwired: 2 in, 2 out]
                            n1561 = property on="light_43" class="Bool (严格)"("Colors [4]"=w702) -> ()  [unwired: 2 in, 2 out]
                            n1562 = property on="light_44" class="Bool (严格)"("Colors [4]"=w701) -> ()  [unwired: 2 in, 2 out]
                            n1563 = property on="light_45" class="Bool (严格)"("Colors [4]"=w700) -> ()  [unwired: 2 in, 2 out]
                            n1564 = property on="light_46" class="Bool (严格)"("Colors [4]"=w699) -> ()  [unwired: 2 in, 2 out]
                            n1565 = property on="light_47" class="Bool (严格)"("Colors [4]"=w698) -> ()  [unwired: 2 in, 2 out]
                            n1566 = property on="light_48" class="Bool (严格)"("Colors [4]"=w697) -> ()  [unwired: 2 in, 2 out]
                          }
                          frame 3 {
                            n1567 = local read "D_IN_4"() -> (w732:string[][])
                            n1568 = Replace Array Subset(array=w732, new element=w731, index (col)=2 ("索引 (列)")) -> (w730:string[][])  [unwired: 1 in]
                            n1569 = Index Array(array=w750, index (row) #1=0 ("索引"), index (row) #2=1 ("索引"), index (row) #3=2 ("索引"), index (row) #4=3 ("索引"), index (row) #5=4 ("索引"), index (row) #6=5 ("索引"), index (row) #7=6 ("索引"), index (row) #8=7 ("索引"), index (row) #9=8 ("索引"), index (row) #10=9 ("索引"), index (row) #11=10 ("索引"), index (row) #12=11 ("索引"), index (row) #13=12 ("索引"), index (row) #14=13 ("索引"), index (row) #15=14 ("索引"), index (row) #16=15 ("索引")) -> (element #1=w749:cluster{u32, u32}[], element #2=w748:cluster{u32, u32}[], element #3=w747:cluster{u32, u32}[], element #4=w746:cluster{u32, u32}[], element #5=w745:cluster{u32, u32}[], element #6=w744:cluster{u32, u32}[], element #7=w743:cluster{u32, u32}[], element #8=w742:cluster{u32, u32}[], element #9=w741:cluster{u32, u32}[], element #10=w740:cluster{u32, u32}[], element #11=w739:cluster{u32, u32}[], element #12=w738:cluster{u32, u32}[], element #13=w737:cluster{u32, u32}[], element #14=w736:cluster{u32, u32}[], element #15=w735:cluster{u32, u32}[], element #16=w734:cluster{u32, u32}[])  [unwired: 16 in]
                            n1570 = local write "D_IN_4"(w730) -> ()
                            n1571 = property on="light_49" class="Bool (严格)"("Colors [4]"=w749) -> ()  [unwired: 2 in, 2 out]
                            n1572 = property on="light_50" class="Bool (严格)"("Colors [4]"=w748) -> ()  [unwired: 2 in, 2 out]
                            n1573 = property on="light_51" class="Bool (严格)"("Colors [4]"=w747) -> ()  [unwired: 2 in, 2 out]
                            n1574 = property on="light_52" class="Bool (严格)"("Colors [4]"=w746) -> ()  [unwired: 2 in, 2 out]
                            n1575 = property on="light_53" class="Bool (严格)"("Colors [4]"=w745) -> ()  [unwired: 2 in, 2 out]
                            n1576 = property on="light_54" class="Bool (严格)"("Colors [4]"=w744) -> ()  [unwired: 2 in, 2 out]
                            n1577 = property on="light_55" class="Bool (严格)"("Colors [4]"=w743) -> ()  [unwired: 2 in, 2 out]
                            n1578 = property on="light_56" class="Bool (严格)"("Colors [4]"=w742) -> ()  [unwired: 2 in, 2 out]
                            n1579 = property on="light_57" class="Bool (严格)"("Colors [4]"=w741) -> ()  [unwired: 2 in, 2 out]
                            n1580 = property on="light_58" class="Bool (严格)"("Colors [4]"=w740) -> ()  [unwired: 2 in, 2 out]
                            n1581 = property on="light_59" class="Bool (严格)"("Colors [4]"=w739) -> ()  [unwired: 2 in, 2 out]
                            n1582 = property on="light_60" class="Bool (严格)"("Colors [4]"=w738) -> ()  [unwired: 2 in, 2 out]
                            n1583 = property on="light_61" class="Bool (严格)"("Colors [4]"=w737) -> ()  [unwired: 2 in, 2 out]
                            n1584 = property on="light_62" class="Bool (严格)"("Colors [4]"=w736) -> ()  [unwired: 2 in, 2 out]
                            n1585 = property on="light_63" class="Bool (严格)"("Colors [4]"=w735) -> ()  [unwired: 2 in, 2 out]
                            n1586 = property on="light_64" class="Bool (严格)"("Colors [4]"=w734) -> ()  [unwired: 2 in, 2 out]
                          }
                          frame 4 {
                            n1587 = local read "D_IN_5"() -> (w769:string[][])
                            n1588 = Replace Array Subset(array=w769, new element=w767, index (col)=2 ("索引 (列)")) -> (w768:string[][])  [unwired: 1 in]
                            n1589 = Index Array(array=w787, index (row) #1=0 ("索引"), index (row) #2=1 ("索引"), index (row) #3=2 ("索引"), index (row) #4=3 ("索引"), index (row) #5=4 ("索引"), index (row) #6=5 ("索引"), index (row) #7=6 ("索引"), index (row) #8=7 ("索引"), index (row) #9=8 ("索引"), index (row) #10=9 ("索引"), index (row) #11=10 ("索引"), index (row) #12=11 ("索引"), index (row) #13=12 ("索引"), index (row) #14=13 ("索引"), index (row) #15=14 ("索引"), index (row) #16=15 ("索引")) -> (element #1=w786:cluster{u32, u32}[], element #2=w785:cluster{u32, u32}[], element #3=w784:cluster{u32, u32}[], element #4=w783:cluster{u32, u32}[], element #5=w782:cluster{u32, u32}[], element #6=w781:cluster{u32, u32}[], element #7=w780:cluster{u32, u32}[], element #8=w779:cluster{u32, u32}[], element #9=w778:cluster{u32, u32}[], element #10=w777:cluster{u32, u32}[], element #11=w776:cluster{u32, u32}[], element #12=w775:cluster{u32, u32}[], element #13=w774:cluster{u32, u32}[], element #14=w773:cluster{u32, u32}[], element #15=w772:cluster{u32, u32}[], element #16=w771:cluster{u32, u32}[])  [unwired: 16 in]
                            n1590 = local write "D_IN_5"(w768) -> ()
                            n1591 = property on="light_65" class="Bool (严格)"("Colors [4]"=w786) -> ()  [unwired: 2 in, 2 out]
                            n1592 = property on="light_66" class="Bool (严格)"("Colors [4]"=w785) -> ()  [unwired: 2 in, 2 out]
                            n1593 = property on="light_67" class="Bool (严格)"("Colors [4]"=w784) -> ()  [unwired: 2 in, 2 out]
                            n1594 = property on="light_68" class="Bool (严格)"("Colors [4]"=w783) -> ()  [unwired: 2 in, 2 out]
                            n1595 = property on="light_69" class="Bool (严格)"("Colors [4]"=w782) -> ()  [unwired: 2 in, 2 out]
                            n1596 = property on="light_70" class="Bool (严格)"("Colors [4]"=w781) -> ()  [unwired: 2 in, 2 out]
                            n1597 = property on="light_71" class="Bool (严格)"("Colors [4]"=w780) -> ()  [unwired: 2 in, 2 out]
                            n1598 = property on="light_72" class="Bool (严格)"("Colors [4]"=w779) -> ()  [unwired: 2 in, 2 out]
                            n1599 = property on="light_73" class="Bool (严格)"("Colors [4]"=w778) -> ()  [unwired: 2 in, 2 out]
                            n1600 = property on="light_74" class="Bool (严格)"("Colors [4]"=w777) -> ()  [unwired: 2 in, 2 out]
                            n1601 = property on="light_75" class="Bool (严格)"("Colors [4]"=w776) -> ()  [unwired: 2 in, 2 out]
                            n1602 = property on="light_76" class="Bool (严格)"("Colors [4]"=w775) -> ()  [unwired: 2 in, 2 out]
                            n1603 = property on="light_77" class="Bool (严格)"("Colors [4]"=w774) -> ()  [unwired: 2 in, 2 out]
                            n1604 = property on="light_78" class="Bool (严格)"("Colors [4]"=w773) -> ()  [unwired: 2 in, 2 out]
                            n1605 = property on="light_79" class="Bool (严格)"("Colors [4]"=w772) -> ()  [unwired: 2 in, 2 out]
                            n1606 = property on="light_80" class="Bool (严格)"("Colors [4]"=w771) -> ()  [unwired: 2 in, 2 out]
                          }
                          frame 1 {
                            n1607 = local read "D_IN_2"() -> (w806:string[][])
                            n1608 = Replace Array Subset(array=w806, new element=w804, index (col)=2 ("索引 (列)")) -> (w805:string[][])  [unwired: 1 in]
                            n1609 = Index Array(array=w824, index (row) #1=0 ("索引"), index (row) #2=1 ("索引"), index (row) #3=2 ("索引"), index (row) #4=3 ("索引"), index (row) #5=4 ("索引"), index (row) #6=5 ("索引"), index (row) #7=6 ("索引"), index (row) #8=7 ("索引"), index (row) #9=8 ("索引"), index (row) #10=9 ("索引"), index (row) #11=10 ("索引"), index (row) #12=11 ("索引"), index (row) #13=12 ("索引"), index (row) #14=13 ("索引"), index (row) #15=14 ("索引"), index (row) #16=15 ("索引")) -> (element #1=w823:cluster{u32, u32}[], element #2=w822:cluster{u32, u32}[], element #3=w821:cluster{u32, u32}[], element #4=w820:cluster{u32, u32}[], element #5=w819:cluster{u32, u32}[], element #6=w818:cluster{u32, u32}[], element #7=w817:cluster{u32, u32}[], element #8=w816:cluster{u32, u32}[], element #9=w815:cluster{u32, u32}[], element #10=w814:cluster{u32, u32}[], element #11=w813:cluster{u32, u32}[], element #12=w812:cluster{u32, u32}[], element #13=w811:cluster{u32, u32}[], element #14=w810:cluster{u32, u32}[], element #15=w809:cluster{u32, u32}[], element #16=w808:cluster{u32, u32}[])  [unwired: 16 in]
                            n1610 = local write "D_IN_2"(w805) -> ()
                            n1611 = property on="light_17" class="Bool (严格)"("Colors [4]"=w823) -> ()  [unwired: 2 in, 2 out]
                            n1612 = property on="light_18" class="Bool (严格)"("Colors [4]"=w822) -> ()  [unwired: 2 in, 2 out]
                            n1613 = property on="light_19" class="Bool (严格)"("Colors [4]"=w821) -> ()  [unwired: 2 in, 2 out]
                            n1614 = property on="light_20" class="Bool (严格)"("Colors [4]"=w820) -> ()  [unwired: 2 in, 2 out]
                            n1615 = property on="light_21" class="Bool (严格)"("Colors [4]"=w819) -> ()  [unwired: 2 in, 2 out]
                            n1616 = property on="light_22" class="Bool (严格)"("Colors [4]"=w818) -> ()  [unwired: 2 in, 2 out]
                            n1617 = property on="light_23" class="Bool (严格)"("Colors [4]"=w817) -> ()  [unwired: 2 in, 2 out]
                            n1618 = property on="light_24" class="Bool (严格)"("Colors [4]"=w816) -> ()  [unwired: 2 in, 2 out]
                            n1619 = property on="light_25" class="Bool (严格)"("Colors [4]"=w815) -> ()  [unwired: 2 in, 2 out]
                            n1620 = property on="light_26" class="Bool (严格)"("Colors [4]"=w814) -> ()  [unwired: 2 in, 2 out]
                            n1621 = property on="light_27" class="Bool (严格)"("Colors [4]"=w813) -> ()  [unwired: 2 in, 2 out]
                            n1622 = property on="light_28" class="Bool (严格)"("Colors [4]"=w812) -> ()  [unwired: 2 in, 2 out]
                            n1623 = property on="light_29" class="Bool (严格)"("Colors [4]"=w811) -> ()  [unwired: 2 in, 2 out]
                            n1624 = property on="light_30" class="Bool (严格)"("Colors [4]"=w810) -> ()  [unwired: 2 in, 2 out]
                            n1625 = property on="light_31" class="Bool (严格)"("Colors [4]"=w809) -> ()  [unwired: 2 in, 2 out]
                            n1626 = property on="light_32" class="Bool (严格)"("Colors [4]"=w808) -> ()  [unwired: 2 in, 2 out]
                          }
                        }
                      }
                    }
                  }
                }
              }
            }
            n1627 = case shown="真" w583 {
              frame False {
              }
              frame True {
                n1628 = call "显示对话框信息3"("Message"="数字量输出数值修改超时") -> ("结束"=w585:bool)  [unwired: 9 in, 1 out]
                n1629 = case shown="真" w585 {
                  frame False {
                  }
                  frame True {
                    n1630 = local write "同步_A1"(5 ("同步_A1")) -> ()
                    n1631 = local write "保持输出"(FALSE ("保持输出")) -> ()
                  }
                }
              }
            }
            n1632 = case shown="真" w584 {
              frame False {
              }
              frame True {
                n1633 = call "显示对话框信息2"("Message"="数字量输出数值修改失败") -> ("结束"=w589:bool)  [unwired: 9 in, 1 out]
                n1634 = case shown="真" w589 {
                  frame False {
                  }
                  frame True {
                    n1635 = local write "同步_A1"(5 ("同步_A1")) -> ()
                    n1636 = local write "保持输出"(FALSE ("保持输出")) -> ()
                  }
                }
              }
            }
          }
          frame #1 {
            n1637 = local read "保持输出"() -> (w843:bool)
            n1638 = case shown="假" w843 {
              frame False {
                n1639 = local read "同步_A2"() -> (w844:i32)
                n1640 = Increment(x=w844) -> (x+1=w845:i32)
                n1641 = local write "同步_A2"(w845) -> ()
              }
              frame True {
              }
            }
          }
        }
      }
    }
    n1642 = local read "关闭？"() -> (w568:bool)
  }
  n1643 = Release Notifier(notifier=w2, error in (no error)=w1) -> ()  [unwired: 1 in, 3 out]
